vi "Dashboard Main.vi"() -> ()   [LabVIEW 2020]
uses:
  <vilib>/Utility/miscctls.llb/LVRectTypeDef.ctl
  <vilib>/event_ctls.llb/eventvkey.ctl
  <vilib>/Rock Robotics/WPI/DriverStation/WPI_DriverStationAllianceInfo.ctl
  <vilib>/Utility/miscctls.llb/LV3DPointTypeDef.ctl
  <vilib>/robotics/Kinematics/DH Kinematic Parameters.ctl
  <vilib>/robotics/Kinematics/Link/Joint Type.ctl
  b1c29fd4-b69e-4c47-bd92-218700034153.vi
  efc637a3-a7e0-4d6a-acb3-aee6468bd1cb.vi
  b2059994-562a-4507-8104-e4c00853bec9.vi
  7fc597ec-ac8e-4325-b133-71466b1fbbcb.vi
  9cac3b8b-4a3f-4d18-bfb1-3aae72e664f2.vi
  a7551b2b-ce58-4830-98e7-c5cf61f6feb4.vi
  cd51690b-7cbe-44fb-a5f0-3232adb0ed53.vi
  a4e8d5d1-2ec3-4e81-be0b-60391cc68073.vi
  dc64ebe6-91bd-4cd7-a1c2-6d709789b2ed.vi
  76b087ca-de3d-4263-8b5c-e25a6bef634b.vi
  1b78be80-bab2-445d-a3e8-82f142a16380.vi
  9e807339-2903-4f51-8fcc-64b6a9381567.vi
  e75f20ac-3dfa-4544-8614-4803d6d17fbb.vi
  273c17a0-a238-4f2a-a55a-7e29d73850ff.vi
  87bdd142-1820-4e26-8582-f713a5f3da40.vi
  b8451b18-7b16-4e07-a196-a1bebf8ce026.vi
  5d307e9f-edd0-4132-a387-09c5916d43b1.vi
  0137daef-9682-45ba-80b9-2d4fda8852b8.vi
  f6a63fab-964b-4051-8314-d4414a0a258c.vi
  90e0fe9d-42b1-4a72-a6c8-4b9d9b3a5a2a.vi
  f15e925d-3118-43e3-bf67-a1272bbf81dd.vi
  394886aa-4cdd-4740-8681-89e3e438764a.vi
  77a42c1f-99bf-4bb6-8218-45b49017f7dc.vi
  5abae45b-ab2b-4816-ba0c-2a0b218f6531.vi
  31f70c1d-3051-4c77-9544-a691198ba614.vi
  f63f5451-5db6-487e-bc86-5cb81e92b132.vi
  81d0db6a-d68a-45c3-b3b1-458879412541.vi
  c235c188-eb56-46fb-93d3-e8acf396af31.vi
  115ba94a-0b26-47fa-ae73-5ec5bd9e502a.vi
  2422668c-951b-48e5-9bda-0f59c56d9c0d.vi
  7776664e-4af7-4b3d-b288-2266642a045e.vi
  6004ed5d-dfc4-4dad-95c1-8e371ea2b9cd.vi
  321ce103-7778-4bb1-9ecc-75a76fef05e9.vi
  d30e88cc-5e2b-4867-b271-53fc6d5cd4d7.vi
  fde90579-e212-4b8a-8145-a17c3e40bcbd.vi
  6c63589b-432e-4f9c-bacb-2063ed7bd576.vi
  b7dcf304-99f6-4f78-9d14-19aa8d9ea562.vi
  e8b3bb93-ba91-445b-94c6-9e998421f827.vi
  0480a820-69ef-45e6-a9f4-d7ff60c89e45.vi
  1c99237e-ea3d-4ecf-b7c2-61034db3ecd2.vi
  58c381f4-7755-468c-a50e-7cea281bf291.vi
  4681331b-9a70-4b27-b9d4-a17199d3c64e.vi
  7eff148d-a456-4b5f-9b0b-1967e164dc83.vi
  7f162a9b-0cf5-4928-819b-a88ae877a425.vi
  748c1db2-33d9-4a44-b6de-b54d4bfa6e8e.vi
  0d2f8b8f-8dae-480e-9309-747785a3eba2.vi
  6da817f6-1561-45f8-a0fe-2c1e5adf6540.vi
  c02c89a6-b8c9-4f9c-9e24-ceb1b894960a.vi
  0a8fe2ab-d060-4915-a9b5-d8978247e2b6.vi
  b1c29fd4-b69e-4c47-bd92-218700034153.vi/77c742ae-e671-49bb-a825-a6e8cebc9f63.vi
  b2059994-562a-4507-8104-e4c00853bec9.vi/77c742ae-e671-49bb-a825-a6e8cebc9f63.vi
  9cac3b8b-4a3f-4d18-bfb1-3aae72e664f2.vi/77c742ae-e671-49bb-a825-a6e8cebc9f63.vi
  a7551b2b-ce58-4830-98e7-c5cf61f6feb4.vi/77c742ae-e671-49bb-a825-a6e8cebc9f63.vi
  cd51690b-7cbe-44fb-a5f0-3232adb0ed53.vi/77c742ae-e671-49bb-a825-a6e8cebc9f63.vi
  a4e8d5d1-2ec3-4e81-be0b-60391cc68073.vi/77c742ae-e671-49bb-a825-a6e8cebc9f63.vi
  dc64ebe6-91bd-4cd7-a1c2-6d709789b2ed.vi/77c742ae-e671-49bb-a825-a6e8cebc9f63.vi
  76b087ca-de3d-4263-8b5c-e25a6bef634b.vi/77c742ae-e671-49bb-a825-a6e8cebc9f63.vi
  1b78be80-bab2-445d-a3e8-82f142a16380.vi/77c742ae-e671-49bb-a825-a6e8cebc9f63.vi
  9e807339-2903-4f51-8fcc-64b6a9381567.vi/77c742ae-e671-49bb-a825-a6e8cebc9f63.vi
  e75f20ac-3dfa-4544-8614-4803d6d17fbb.vi/77c742ae-e671-49bb-a825-a6e8cebc9f63.vi
  0137daef-9682-45ba-80b9-2d4fda8852b8.vi/77c742ae-e671-49bb-a825-a6e8cebc9f63.vi
  f6a63fab-964b-4051-8314-d4414a0a258c.vi/77c742ae-e671-49bb-a825-a6e8cebc9f63.vi
  90e0fe9d-42b1-4a72-a6c8-4b9d9b3a5a2a.vi/77c742ae-e671-49bb-a825-a6e8cebc9f63.vi
  f15e925d-3118-43e3-bf67-a1272bbf81dd.vi/77c742ae-e671-49bb-a825-a6e8cebc9f63.vi
  394886aa-4cdd-4740-8681-89e3e438764a.vi/77c742ae-e671-49bb-a825-a6e8cebc9f63.vi
  77a42c1f-99bf-4bb6-8218-45b49017f7dc.vi/77c742ae-e671-49bb-a825-a6e8cebc9f63.vi
  5abae45b-ab2b-4816-ba0c-2a0b218f6531.vi/77c742ae-e671-49bb-a825-a6e8cebc9f63.vi
  31f70c1d-3051-4c77-9544-a691198ba614.vi/77c742ae-e671-49bb-a825-a6e8cebc9f63.vi
  f63f5451-5db6-487e-bc86-5cb81e92b132.vi/77c742ae-e671-49bb-a825-a6e8cebc9f63.vi
  81d0db6a-d68a-45c3-b3b1-458879412541.vi/77c742ae-e671-49bb-a825-a6e8cebc9f63.vi
  c235c188-eb56-46fb-93d3-e8acf396af31.vi/77c742ae-e671-49bb-a825-a6e8cebc9f63.vi
  115ba94a-0b26-47fa-ae73-5ec5bd9e502a.vi/77c742ae-e671-49bb-a825-a6e8cebc9f63.vi
  2422668c-951b-48e5-9bda-0f59c56d9c0d.vi/77c742ae-e671-49bb-a825-a6e8cebc9f63.vi
  7776664e-4af7-4b3d-b288-2266642a045e.vi/77c742ae-e671-49bb-a825-a6e8cebc9f63.vi
  6004ed5d-dfc4-4dad-95c1-8e371ea2b9cd.vi/77c742ae-e671-49bb-a825-a6e8cebc9f63.vi
  321ce103-7778-4bb1-9ecc-75a76fef05e9.vi/77c742ae-e671-49bb-a825-a6e8cebc9f63.vi
  d30e88cc-5e2b-4867-b271-53fc6d5cd4d7.vi/77c742ae-e671-49bb-a825-a6e8cebc9f63.vi
  fde90579-e212-4b8a-8145-a17c3e40bcbd.vi/77c742ae-e671-49bb-a825-a6e8cebc9f63.vi
  6c63589b-432e-4f9c-bacb-2063ed7bd576.vi/77c742ae-e671-49bb-a825-a6e8cebc9f63.vi
  b7dcf304-99f6-4f78-9d14-19aa8d9ea562.vi/77c742ae-e671-49bb-a825-a6e8cebc9f63.vi
  e8b3bb93-ba91-445b-94c6-9e998421f827.vi/77c742ae-e671-49bb-a825-a6e8cebc9f63.vi
  0480a820-69ef-45e6-a9f4-d7ff60c89e45.vi/77c742ae-e671-49bb-a825-a6e8cebc9f63.vi
  1c99237e-ea3d-4ecf-b7c2-61034db3ecd2.vi/77c742ae-e671-49bb-a825-a6e8cebc9f63.vi
  58c381f4-7755-468c-a50e-7cea281bf291.vi/77c742ae-e671-49bb-a825-a6e8cebc9f63.vi
  4681331b-9a70-4b27-b9d4-a17199d3c64e.vi/77c742ae-e671-49bb-a825-a6e8cebc9f63.vi
  7eff148d-a456-4b5f-9b0b-1967e164dc83.vi/77c742ae-e671-49bb-a825-a6e8cebc9f63.vi
  7f162a9b-0cf5-4928-819b-a88ae877a425.vi/77c742ae-e671-49bb-a825-a6e8cebc9f63.vi
  748c1db2-33d9-4a44-b6de-b54d4bfa6e8e.vi/77c742ae-e671-49bb-a825-a6e8cebc9f63.vi
  0d2f8b8f-8dae-480e-9309-747785a3eba2.vi/77c742ae-e671-49bb-a825-a6e8cebc9f63.vi
  <vilib>/robotics/Kinematics/RotateX.vi
  <vilib>/robotics/Kinematics/RotateY.vi
  <vilib>/robotics/Kinematics/RotateZ.vi
  <vilib>/Analysis/baseanly.llb/A x B.vi
  <vilib>/Analysis/baseanly.llb/Real A x B.vi
  0a8fe2ab-d060-4915-a9b5-d8978247e2b6.vi/77c742ae-e671-49bb-a825-a6e8cebc9f63.vi
  <vilib>/Utility/xml.llb/Read From XML File(array).vi
  <vilib>/Utility/xml.llb/Write to XML File(string).vi
  <vilib>/Rock Robotics/Network Tables/NT Read Number.vi
  <vilib>/Rock Robotics/Network Tables/NT Read Boolean.vi
  GlobalDashboard.vi
  <vilib>/Rock Robotics/Network Tables/NT Read String.vi
  <vilib>/Rock Robotics/Network Tables/NT Write Number.vi
  <vilib>/Rock Robotics/Network Tables/NT Read Numeric Array.vi
  <vilib>/Rock Robotics/Network Tables/NT Write Boolean.vi
  <vilib>/Rock Robotics/Network Tables/NT Read String Array.vi
  <vilib>/Rock Robotics/Network Tables/NT Read Boolean Array.vi
  <vilib>/Rock Robotics/Network Tables/NT Write String.vi
  <vilib>/Rock Robotics/Network Tables/NT Write Numeric Array.vi
  <vilib>/robotics/Kinematics/Analytical/Initialize Generic Serial Arm.vi
  <vilib>/picture/3D Picture Control/Object/Create Object (drawable).vi
  <vilib>/picture/3D Picture Control/Object/Add Object (no reference).vi
  <vilib>/Rock Robotics/Network Tables/NT Write String Array.vi
  <vilib>/vision/NI_Vision_Development_Module.lvlib
  <vilib>/picture/3D Picture Control/NI_3D Picture Control.lvlib
  <vilib>/robotics/Kinematics/Plotting/NI_Robotics_3DKinematics.lvlib
  <vilib>/robotics/Kinematics/Robot/NI_Robotics_Serial Robot Arm.lvclass
  <vilib>/robotics/Kinematics/Analytical/NI_Robotics_AnalyticKinematics.lvlib
  <vilib>/robotics/Kinematics/Link/NI_Robotics_Link.lvclass
  <vilib>/robotics/Kinematics/NI_Kinematics.lvlib
panel:
  in  "TCP":refnum<k5>
  in  "Dashboard Tab":T1(tab)=enum."Setup/Auto"
  in  "CheckList":i32(listbox)
  in  "Apply_Grid_Calibration":bool
  out "Current_Red_Calibration":dbl format="%.1f"
  in  "New_Red_Calibration":dbl format="%.1f"
  out "Heading_to_Target":dbl format="%.1f"
  out "Distance_to_Target":dbl format="%.1f"
  out "Robot_P":dbl format="%.1f"
  in  "Enable_Streaming_GUI":bool=TRUE
  out "Robot_Profile_GUI":string
  out "Auto_Playbook_GUI":string
  in  "Select Driver Profile":u16(ring) items=["N/A"]
  in  "Camera Name":string(combo)="limelight"
  in  "Camera Settings":T2={"Frame Rate"=20, "Compression"=60, "Size"=1, "DB Camera Config"=FALSE} {"Size" items=["640x480", "320x240", "160x120"]}
  in  "Select Autonomous Play":u16(ring) items=["N/A"]
  out "Master_Caution_GUI_0":bool caption="Mode_Butterfly"
  out "Robot_is_Autonomous_GUI_0":bool caption="Mode_Butterfly"
  out "Robot_Code_Version_GUI":string
  out "Auto_Suffix_GUI":string
  in  "Refresh_Auto_Play_List_GUI":bool
  in  "Auto_Delay_GUI":dbl format="%.1f"
  in  "Manual_Start_X":dbl min=0.0 max=700.0 format="%.1f"
  out "Robot_X":dbl format="%.1f"
  out "Robot_Y":dbl format="%.1f"
  in  "Manual_Start_Y":dbl min=0.0 max=400.0 format="%.1f"
  out "Robot_H_GUI":dbl format="%.1f"
  in  "Manual_Start_H":dbl min=0.0 max=360.0 format="%.1f"
  in  "Field Map":u16(ring) items=["N/A"]
  in  "Push_Robot_Start_GUI":bool
  in  "Export_Robot_Pose":bool
  in  "Clear_Robot_Pose_Display":bool
  in  "Dock_Dashboard":bool
  in  "Force_Human_Control_GUI":bool
  in  "Auto_Test_Mode_GUI":bool
  in  "Disable_Fusion_While_Autonomous":bool
  in  "Disable_Fusion_While_Disabled":bool=TRUE
  out "Robot Pose 1":cluster{dbl[], dbl[]}[](graph)
  in  "New_Blue_Calibration":dbl format="%.1f"
  out "Current_Blue_Calibration":dbl format="%.1f"
  in  "Scoring Position":u16(ring) items=["MID", "HIGH"]
  in  "TeleOp Starting State":u16(ring) items=["STOW", "GROUND"]
  out "Help Graphic":T3(plugin-control)
  out "Hybrid_Node_Names":bool
  out "Scored_Hybrid_Nodes":bool[](array[boolean])
  out "Nearest_Hybrid_Node":bool[](array[boolean])
  out "LL_Ret_Left":bool
  out "LL_Ret_Right":bool
  out "WA_Ret_Right":bool
  out "WA_Ret_Left":bool
  out "Gripper_Motor_Fault":bool
  out "Gripper_Overheating":bool
  out "Swerve_Drive_Fault":bool
  out "Arm_Motor_Over_Current":bool
  out "Arm_Motor_Fault":bool
  out "State_Score":bool
  out "State_Shelf":bool
  in  "Arm_Override":bool
  out "Score_State_LVL2_Indicator":bool
  out "Score_State_LVL1_Indicator":bool
  out "Arm_Overheating":bool
  out "Robot Pose 2":cluster{dbl[], dbl[]}[](graph)
  out "Master_State_SHLF_Indicator":bool
  out "Master_State_GRND_Indicator":bool
  out "Master_State_HOPR_Indicator":bool
  out "Master_State_SCOR_Indicator":bool
  out "Master_State_BLNC_Indicator":bool
  out "Master_State_STOW_Indicator":bool
  out "Vision_Fault_GUI":bool
  out "Pressure_Leak_GUI":bool
  in  "Master_Safety_Override_1":bool
  in  "Manipulator_Help":bool
  in  "Driver_Help":bool
  out "No_Secondary_Camera":bool
  out "Swerve_Shifter_Failure":bool
  out "Electrical_Fault_GUI":bool
  out "Diverting_Power_GUI":bool
  out "CAN_Bus_Fault_GUI":bool
  out "IMU_Failure_GUI":bool
  out "Robot_is_Autonomous_GUI_1":bool caption="Mode_Butterfly"
  out "LL_Valid":bool caption="Mode_Butterfly"
  out "Auto_Error_GUI":bool
  in  "Clear_Errors_GUI":bool
  out "Swerve_Azimuth_Fault":bool
  out "Pressure_Transducer_GUI":dbl(slide) scale=0.0..115.0
  out "Pressure_Vent_GUI":bool
  out "Swerve_Overheating":bool
  out "Compressor_On_GUI":bool
  in  "Right":bool
  in  "Reticule":T4(ring)
  in  "Save":bool
  in  "Up":bool
  in  "Down":bool
  in  "Left":bool
  out "Master_Caution_GUI_1":bool caption="Mode_Butterfly"
  out "Battery_Critical_GUI":bool
  out "Battery_Voltage_GUI":dbl(slide) scale=11.0..13.0
  out "Field_Oriented_GUI":bool caption="Mode_Butterfly"
  out "Slow_Loop":bool
  out "Combined Camera Feed":T3(plugin-control)
  in  "Camera_Override_GUI":bool
  in  "Field_Oriented_Override_GUI":bool
  out "Arm_Has_Arrived":bool caption="Mode_Butterfly"
  out "Pointed_at_Target":bool caption="Mode_Butterfly"
  in  "Auto_Targeting_Override":bool
  out "Arm_Motor_Fault_Array":bool[](array[boolean])
  out "Arm_Motor_Over_Current_Array":bool[](array[boolean])
  out "State_Hopper":bool
  out "Gripper_Outtaking":bool caption="Mode_Butterfly"
  out "Gripper_Intaking":bool caption="Mode_Butterfly"
  out "Gamepiece_Grabbed_1":bool caption="Mode_Butterfly"
  out "Using_Auto_Targeting":bool caption="Mode_Butterfly"
  out "Gripper_Velocity":dbl
  out "Swerve_Output_Loop_Time_GU":u32
  in  "Simulate_Arm":bool
  in  "Jog Z (in)":dbl min=-100.0 max=100.0 step=1.0 format="%.1g"
  in  "Unlock_Arm_Joints":bool
  out "Shoulder_Temp":dbl
  out "Ebow_Temp":dbl
  out "Wrist_Temp":dbl
  in  "Reset 3D View":bool
  out "Swerve_3_Drive_Velocity":dbl format="%.1f"
  out "Swerve_3_Azimuth_Position":dbl format="%.1f"
  out "Swerve_3_Drive_Temperature":dbl
  out "Swerve_0_Drive_Temperature":dbl
  out "Camera Perf":string
  out "Control_Loop_Time_GUI":u32
  in  "Calibrate_Wheels_GUI":bool
  in  "Home_Wheels_GUI":bool
  out "Swerve_0_Azimuth_Position":dbl format="%.1f"
  out "Swerve_0_Drive_Velocity":dbl format="%.1f"
  out "Swerve_1_Drive_Velocity":dbl format="%.1f"
  out "Swerve_1_Azimuth_Position":dbl format="%.1f"
  out "Swerve_1_Drive_Temperature":dbl
  out "Swerve_2_Drive_Velocity":dbl format="%.1f"
  out "Swerve_2_Azimuth_Position":dbl format="%.1f"
  out "Swerve_2_Drive_Temperature":dbl
  in  "Arm_Calibrate_Wheels_GUI":bool
  out "Master_Caution_GUI_2":bool caption="Mode_Butterfly"
  in  "Actuator Testing":u16(ring) items=["N/A"]
  in  "Test_Actuator_Value_GUI":dbl step=0.1 format="%.2f"
  in  "Calibrate_Joysticks_GUI":bool
  in  "Arm_Calibrate_Joysticks":bool
  out "Robot_is_Autonomous_GUI_2":bool caption="Mode_Butterfly"
  in  "Test_Actuator_Period_GUI":dbl min=0.0 step=1.0 format="%.2f"
  out "Pose_Loop_Time_GUI":u32
  in  "Mute_Audible_Warnings":bool
  out "Combined Error String":string
  out "Swerve_0_Shifter_State":string
  out "Swerve_1_Shifter_State":string
  out "Swerve_3_Shifter_State":string
  out "Swerve_2_Shifter_State":string
  out "Swerve_Azimuth_Fault_Array":bool[](array[boolean])
  in  "Super_Test_Mode_GUI":bool
  out "Current_Driver_Profile_Setpoints_GUI":T5={"Strafe Deadband"=0.08, "Strafe Scaling"=2.0, "Strafe Maximum"=0.5, "Rotation Deadband"=0.15, "Rotation Scaling"=2.5, "Rotation Maximum"=0.5} {"Rotation Maximum" min=0.3 max=1.0 scale=0.3..1.0; "Rotation Scaling" min=1.0 max=4.0 scale=1.0..4.0; "Rotation Deadband" min=0.0 max=0.25 scale=0.0..0.25; "Strafe Maximum" min=0.3 max=1.0 scale=0.3..1.0; "Strafe Scaling" min=1.0 max=4.0 scale=1.0..4.0; "Strafe Deadband" min=0.0 max=0.25 scale=0.0..0.25}
  in  "New_Driver_Profile_Setpoints_GUI":T6={"Strafe Deadband"=0.08, "Strafe Scaling"=2.0, "Strafe Max"=0.5, "Rotate Deadband"=0.15, "Rotate Scaling"=2.5, "Rotate Max"=0.5} {"Rotate Max" min=0.3 max=1.0 format="%.2g"; "Rotate Scaling" min=1.0 max=4.0 format="%.2g"; "Rotate Deadband" min=0.0 max=0.25 format="%.2g"; "Strafe Max" min=0.3 max=1.0 format="%.2g"; "Strafe Scaling" min=1.0 max=4.0 format="%.2g"; "Strafe Deadband" min=0.0 max=0.25 format="%.2g"}
  in  "Apply_Driver_Profile_Setpoints_GUI":bool
  out "Current_Driver_Profile_GUI":string
  in  "Free_Tuning_Variable_GUI":dbl min=0.0 step=1.0 format="%.3f"
  out "Audible_Warnings_Enabled_GUI":bool
  out "Legal_Drivers_GUI":string[](array[string])
  out "Swerve_Shifter_Failure_Array":bool[](array[boolean])
  out "Swerve_Overheating_Array":bool[](array[boolean])
  out "3D Arm Model":refnum<vi>(3d-picture)
  out "Shoulder_Current_Angle":dbl format="%.1f"
  out "Ebow_Current_Angle":dbl format="%.1f"
  out "Wrist_Current_Angle":dbl format="%.1f"
  out "Arm_Overheating_Array":bool[](array[boolean])
  out "Grabbed_Gamepiece_Enum":enum16{"CUBE", "CONE"}(ring)
  in  "Calibrate_Arm":bool
  in  "Arm_Calibrate_Arm":bool
  in  "Jog X (in)":dbl min=-100.0 max=100.0 step=1.0 format="%.1g"
  out "Gamepiece_Grabbed_2":bool caption="Mode_Butterfly"
  out "End_Effector_X":dbl format="%.1f"
  out "End_Effector_Z":dbl format="%.1f"
  out "Swerve_Drive_Fault_Array":bool[](array[boolean])
  out "Gripper_Temperature":dbl
  out "NT Connection":bool
  out "Mode":T7(ring)=enum."Auto Disabled"
  out "Tree":string(tree)
  out "Background":bool
  # "2023 Dashboard v2.3-dev"
  # "Robot Profile"
  # "Robot X Position (in)"
  # "Robot Y Position (in)"
  # "Delay (s)"
  # "Suffix"
  # "X (in)"
  # "Robot Heading (deg)"
  # "Autonomous Playbook Entry"
  # "Robot Pitch (deg)"
  # "Auto Test\nMode"
  # "Force\nHuman"
  # "Y (in)"
  # "Target Distance (in)"
  # "H (deg)"
  # "Target Heading (deg)"
  # "Undock Dashboard"
  # "Yes Camera Streaming"
  # "Stop Fusion While Auto"
  # "Stop Fusion While Disabled"
  # "Grid Y Calibration (in)"
  # "X"
  # "Y"
  # "MASTER\nSTATES"
  # "OVERRIDES"
  # "Camera Override"
  # "Robot-Oriented Drive Controls"
  # "Arm Motion Override"
  # "Auto-Targeting Override"
  # "SCORE\nSTATES"
  # "Disengage\nSafeties"
  # "11"
  # "13"
  # "0"
  # "120"
  # "Drivebase Subsytem"
  # "Arm and Gripper Subsytems"
  # "Driver Profile Selected"
  # "Calibrate Arm Encoders"
  # "Loop Times"
  # "Module 1"
  # "Module 0"
  # "Control (ms)"
  # "Azimuth (deg)"
  # "Pose (ms)"
  # "Temp (C)"
  # "Simulate the Arm"
  # "Unlock Arm Joints"
  # "Drive Output (ms)"
  # "Velocity (ft/s)"
  # "Shifter State"
  # "Module 2"
  # "Module 3"
  # "Variable (bleh)"
  # "Disabled\nTest Mode"
  # "Azimuth (deg)"
  # "Temp (C)"
  # "Velocity (ft/s)"
  # "Shifter State"
  # "Calibrate Wheels"
  # "Gripper"
  # "Shoulder"
  # "Elbow"
  # "Wrist"
  # "Period (s)"
  # "Calibrate Joysticks"
  # "Amplitude"
  # "Relative (deg)"
  # "Velocity (rpm)"
  # "Temp (C)"
  # "Temp (C)"
  # "0"
  # "0.25"
  # "1"
  # "4"
  # "0.3"
  # "1"
  # "0"
  # "0.25"
  # "1"
  # "4"
  # "0.3"
  # "1"
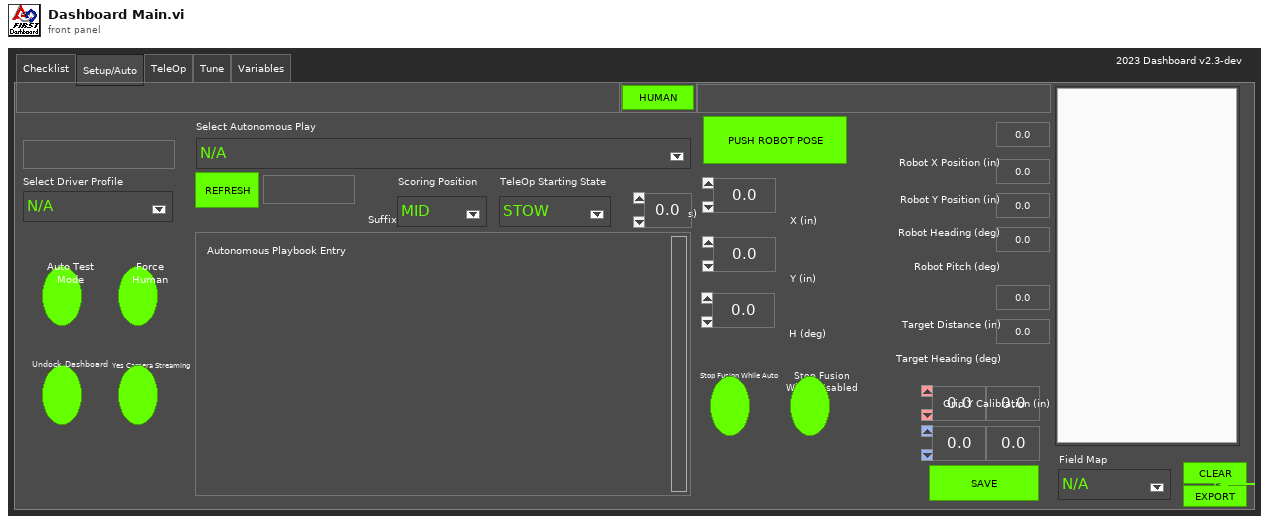
[diagram p1: front panel]
types:
  T1 = enum32{"Checklist", "Setup/Auto", "TeleOp", "Tune", "NT", "Test", "Commands", "Variables"}
  T2 = cluster{"Frame Rate":i32, "Compression":i32, "Size":u16, "DB Camera Config":bool}
  T3 = typedef "IMAQ Image.ctl" = refnum<image>
  T4 = enum16{"Wide Angle Left Reticule", "Wide Angle Right Reticule", "Lime Light Left Reticule", "Lime Light Right Reticule"}
  T5 = cluster{"Strafe Deadband":dbl, "Strafe Scaling":dbl, "Strafe Maximum":dbl, "Rotation Deadband":dbl, "Rotation Scaling":dbl, "Rotation Maximum":dbl}
  T6 = cluster{"Strafe Deadband":dbl, "Strafe Scaling":dbl, "Strafe Max":dbl, "Rotate Deadband":dbl, "Rotate Scaling":dbl, "Rotate Max":dbl}
  T7 = enum8{"Tele-Op Disabled", "Tele-Op Enabled", "Auto Disabled", "Auto Enabled", "Test Disabled", "Test Enabled", "Disconnected", "No Code", "E-Stop"}
  T8 = cluster{"Save Path":path, "Interval (s)":dbl, "Keep":i32}
  T9 = enum32{"Drive", "Camera", "Basic", "Custom", "Test", "Commands", "Checklist", "Variables"}
  T10 = cluster{"IDs":cluster{"RPC field ID":u16, "Unique ID":u16}, "String":string}
  T11 = typedef "Image Type" = u32
  T12 = typedef "WPI_DriverStationAllianceInfo.ctl" = enum16{"Red", "Blue", "Invalid"}
  T13 = typedef "LV3DPointTypeDef.ctl" = cluster{"X":sgl, "Y":sgl, "Z":sgl}
  T14 = cluster{"Red":sgl, "Green":sgl, "Blue":sgl, "Alpha":sgl}
  T15 = enum8{"Enabled", "Disabled", "Disabled and Grayed Out"}
  T16 = cluster{"Error Strings":string, "Disable Counts":cluster{u16, u16}, "Rail Faults":cluster{u16, u16, u16}, "Robot IP":string, "DB Mode":u8, "Event Info":cluster{"Name":string, "Type":u8, "Number":u16, "Replay":u8}}
  T17 = cluster{"Storage":cluster{"Disk Free":u64, "RAM Block":u32, "RAM free":u32}, "CPU Utilization":cluster{"CPU % ISR":sgl, "CPU % Time Crit":sgl, "CPU % Timed Str":sgl, "CPU % High":sgl, "CPU % Above":sgl, "CPU % Normal":sgl, "CPU % Low":sgl}, "CAN":cluster{"% Bus Utilization":sgl, "Bus Off Cnt":u32, "TX_FIFO Full Cnt":u32, "Receive Error Cnt":u8, "Transmit Error Cnt":u8}, "HID":cluster{"HID Outputs":u32, "Rumble Low":u16, "Rumble High":u16}[]}
  T18 = cluster{"Status bits":cluster{"Test Mode":bool, "Autonomous":bool, "Enabled":bool, "Code Start":bool, "Brownout":bool, "Reserved 2":bool, "Reserved 3":bool, "E-Stop":bool}, "Code Trace":cluster{"Disabled":bool, "TeleOp":bool, "Auto":bool, "Test":bool}, "Controller Type":enum16{"unknown", "cRIO", "roboRio"}, "Code?":enum16{"unknown", "noCode", "code"}, "Battery V":dbl}
  T19 = cluster{"Control Bits":cluster{"TestMode":bool, "Autonomous":bool, "Enabled":bool, "FMS Present":bool, bool, bool, bool, "E-Stop":bool}, "Team Station ":u8, "Countdown":sgl, "Joystick Values":cluster{"Axes":dbl[], "Buttons":bool[], "POVs":i16[]}[]}
  T20 = typedef "imagedata.ctl" = cluster{"image type":i32, "image depth":i32, "image":u8[], "mask":u8[], "colors":u32[], "Rectangle":cluster{"left":i16, "top":i16, "right":i16, "bottom":i16}}
  T21 = cluster{"Boolean":bool, "Numeric Text.Text Colors:Text Color":u32}
  T22 = cluster{"value[0]":dbl, "value[1]":dbl, "value[2]":dbl, "value[3]":dbl, "value[4]":dbl, "value[5]":dbl}
  T23 = typedef "DH Kinematic Parameters.ctl" = cluster{"twist angle":dbl, "length":dbl, "rotation angle":dbl, "offset distance":dbl, "joint type":T24, "joint coordinate offset":dbl}
  T24 = typedef "NI_Robotics_Link.lvclass/Joint Type.ctl" = enum16{"Revolute", "Prismatic"}
  T25 = typedef "NI_Matrix.lvlib/RealMatrix.ctl" = dbl[][]
  T26 = cluster{"Numeric":dbl, "Numeric":dbl, "Numeric":dbl}
  T27 = typedef "LVRectTypeDef.ctl" = cluster{"Left":i16, "Top":i16, "Right":i16, "Bottom":i16}
  T28 = typedef "eventvkey.ctl" = enum16{"ASCII", "Enter", "Return", "Shift", "Ctrl", "Alt", "Cmd", "Opt", "Caps", "NumLock", "Clear", "Break", "Up", "Down", "Left", "Right", "Insert", "Delete", "Home", "End", "PageUp", "PageDown", "Escape", "Help", "Pause", "ScrollLock", "F1", "F2", "F3", "F4", "F5", "F6", "F7", "F8", "F9", "F10", "F11", "F12", "F13", "F14", "F15", "F16", "F17", "F18", "F19", "F20", "F21", "F22", "F23", "F24", "Play", "VolumeUp", "VolumeDown", "Mute", "Two Byte Char"}
  T29 = cluster{"Shift":bool, "Ctrl":bool, "Alt":bool, "Cmd":bool, "Opt":bool}
  T30 = cluster{"WA_Ret_Left":refnum<vi>, "WA_Ret_Right":refnum<vi>, "LL_Ret_Left":refnum<vi>, "LL_Ret_Right":refnum<vi>}
  T31 = cluster{"Camera Name":string, string, "Saved DB Images Info":cluster{"Save Path":path, "Interval (s)":dbl, "Keep":i32}}
  T32 = cluster{string, "Arm_Motor_Over_Current":bool, dbl}
  T33 = cluster{string, "Swerve_Shifter_Failure":bool, dbl}
  T34 = cluster{string, "Master_Safety_Override_1":bool, dbl}
  T35 = cluster{string, "Swerve_Azimuth_Fault":bool, dbl}
  T36 = cluster{string, "Arm_Calibrate_Wheels_GUI":bool, dbl}
  T37 = cluster{string, "Electrical_Fault_GUI":bool, dbl}
  T38 = cluster{string, "Arm_Calibrate_Joysticks":bool, dbl}
  T39 = cluster{string, "Gripper_Motor_Fault":bool, dbl}[]
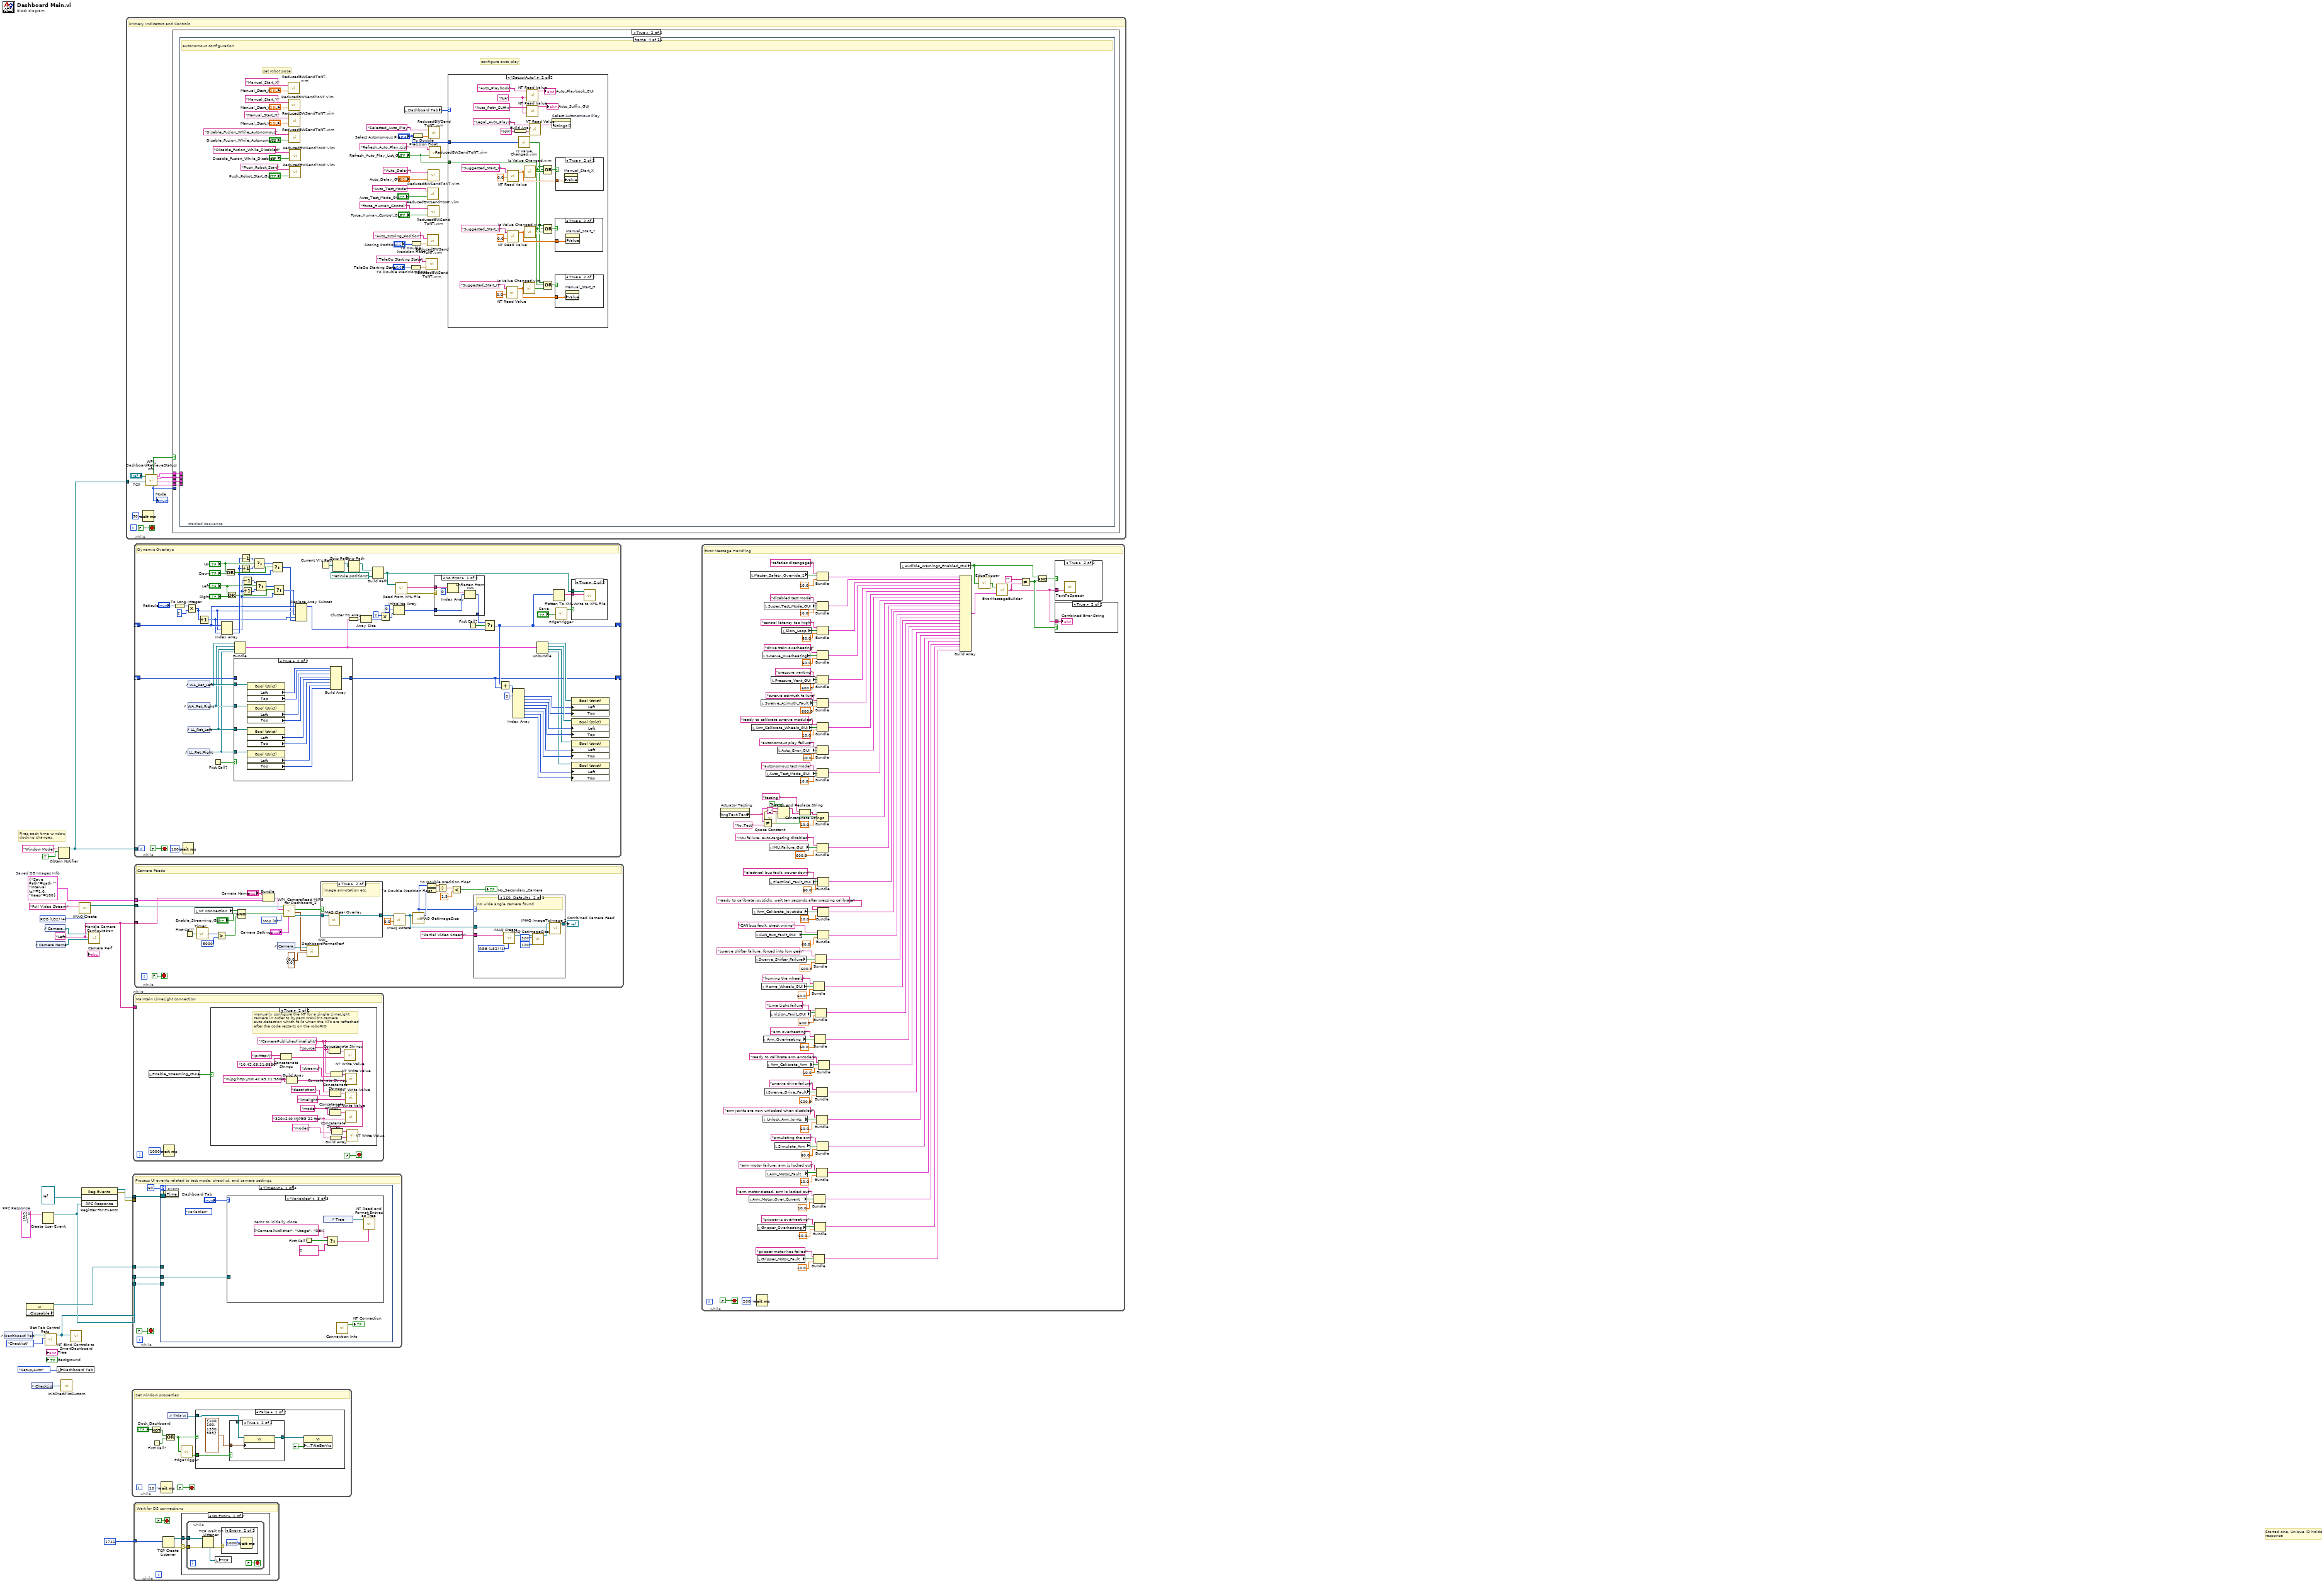
[diagram p0: block diagram]
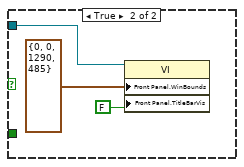
[diagram p4: hidden frame]
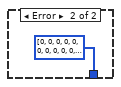
[diagram p7: hidden frame]
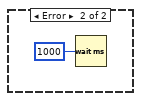
[diagram p11: hidden frame]
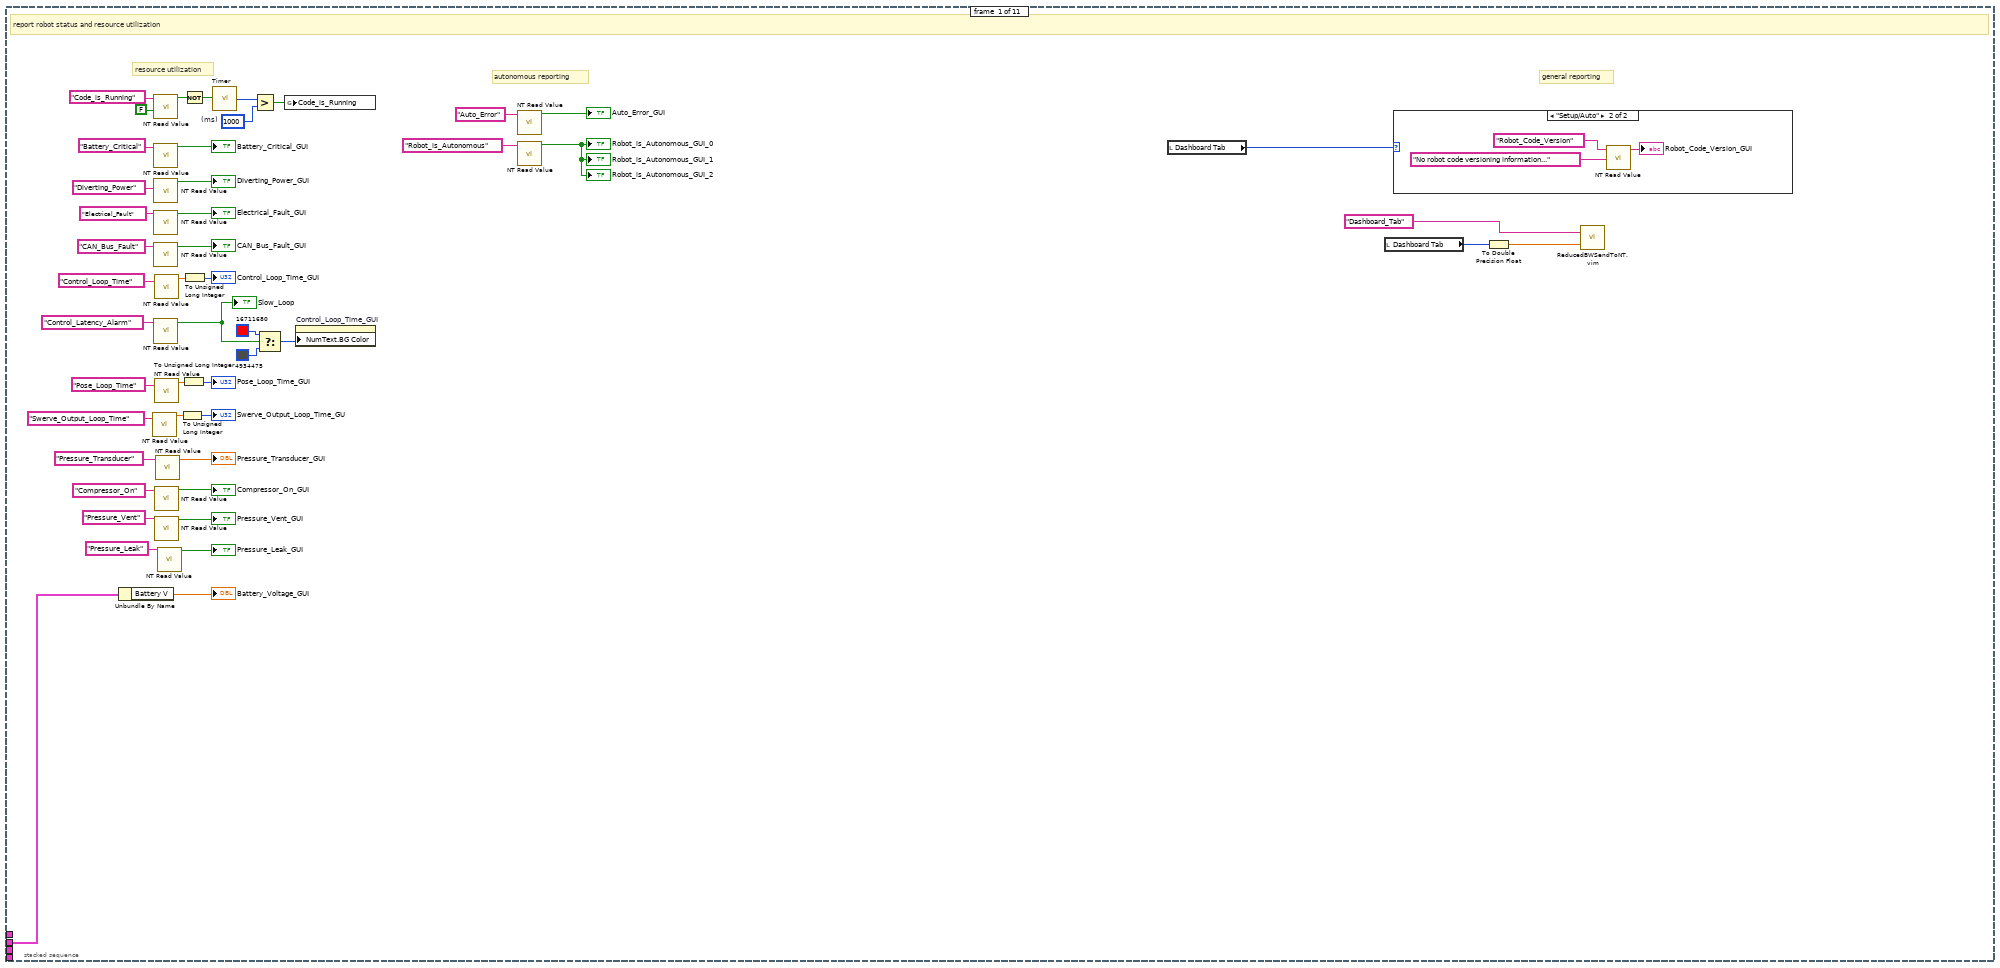
[diagram p13: hidden frame]
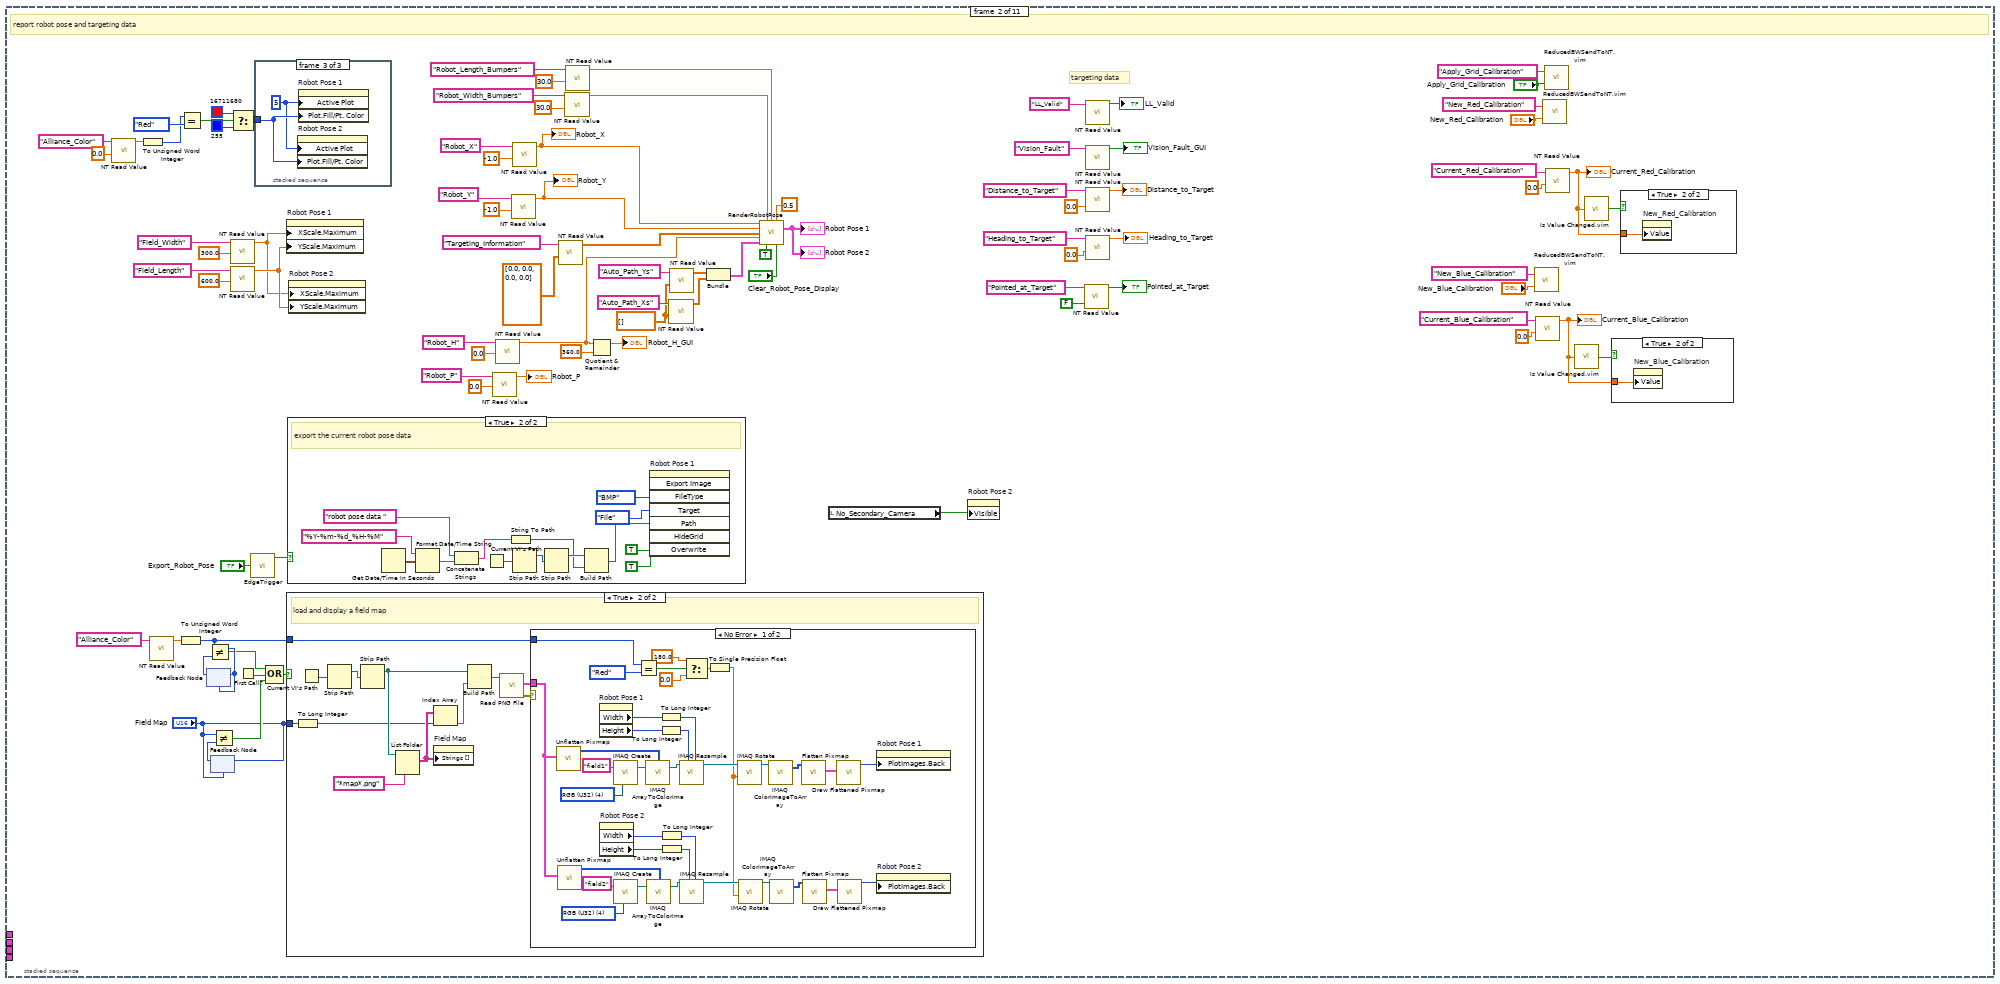
[diagram p15: hidden frame]
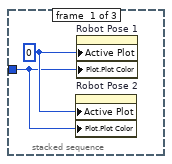
[diagram p18: hidden frame]
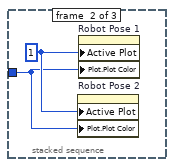
[diagram p19: hidden frame]
diagram:
  w10 = T8 {"Save Path"=path "", "Interval (s)"=1.0, "Keep"=180}  # Saved DB Images Info
  w3 = "Left"
  w13 = T10 {"IDs"={"RPC field ID"=0, "Unique ID"=0}, "String"=""}  # RPC Response
  w6 = T11 4 items=["Grayscale (U8)", "Grayscale (I16)", "Grayscale (SGL)", "Complex (CSG)", "RGB (U32)", "HSL (U32)", "RGB (U64)"] ("Image Type")
  # "Started one, Unique ID holds\nresponse"
  # "Fires each time window\ndocking changes."
  n1 = control-ref of="Dashboard Tab"() -> (w16:refnum<vi>)
  n2 = property class="VI" props=["Front Panel.Closeable"]() -> (reference out=w17:refnum<vi>)  [unwired: 2 in, 2 out]
  n3 = control-ref of="CheckList"() -> (w5:refnum<vi>)
  n4 = control-ref of="Camera Name"() -> (w8:refnum<vi>)
  n5 = Create User Event(user event datatype=w13) -> (user event=w12:refnum<user-event>)  [unwired: 1 in, 1 out]
  n6 = control-ref of="Camera Settings"() -> (w9:refnum<vi>)
  n7 = call <vilib>:"Get Tab Control Refs.vi"("Page Index"=T9."Checklist" ("Dashboard Tab"), "TabControl in"=w16) -> ("ControlsOnPage"=w2:refnum<vi>[])  [unwired: 9 in]
  n8 = local write "Dashboard Tab"(T1."Setup/Auto" ("Dashboard Tab")) -> ()
  n9 = Obtain Notifier(name (unnamed)="Window Mode", notification data type=TRUE) -> (notifier out=w1:refnum<notifier>)  [unwired: 2 in, 2 out]
  n10 = call "InitChecklistCustom.vi"("ListBox in"=w5) -> ()  [unwired: 1 in]
  n11 = call <vilib>:"NT Bind Controls to SmartDashboard.vi"("Bound Control Refs"=w2) -> ()  [unwired: 11 in]
  n12 = call "IMAQ Create"("Image Name"="Full Video Stream", "Image Type"=w6) -> ("New Image"=w4:T3)  [unwired: 2 in, 2 out]
  n13 = register-events(refnum<vi> refnum, w12) -> (reference out=w20:refnum<event-registration>, error out=w19:errorcluster)  [unwired: 2 in]
  n14 = call "Handle Camera Configuration.vi"("CameraNameRef"=w8, "Display Name"=w3, "ClusterRef"=w9) -> ()  [unwired: 9 in]
  n15 = while {
    tunnel: w1 -> [w24]
    stop <- FALSE stop-if-true
    # "Primary Indicators and Controls"
    n16 = Wait (ms)(milliseconds to wait=u32 50) -> ()  [unwired: 1 out]
    n17 = call <vilib>:"WPI_DashboardRetrieveStatusInfo.vi"("Window Mode Notifier"=w24, "TCP Cnx"="TCP") -> ("Power and Errors"=w27:T16, "Robot Metrics"=w30:T17, "Status Info"=w31:T18, "Control Info"=w28:T19, "Robot Mode"=w26:T7, "Process?"=w29:bool)  [unwired: 4 in]
    "Mode" <- w26
    n18 = case shown="True" w29 {
      tunnel: w31 -> [_ w35]
      tunnel: w30 -> [_ w34]
      tunnel: w28 -> [_ w36]
      tunnel: w27 -> [_ w33]
      tunnel: w26 -> [_ _]
      frame False {
      }
      frame True {
        n19 = stacked-sequence {
          tunnel: w36 -> [_ _ _ _ _ _ _ _ _ _ _]
          tunnel: w35 -> [w51 _ _ _ _ _ _ _ _ _ _]
          tunnel: w34 -> [_ _ _ _ _ _ _ _ _ _ _]
          tunnel: w33 -> [_ _ _ _ _ _ _ _ _ _ _]
          frame #0 {
            w41 = u32 1000  # (ms)
            # "general reporting"
            # "resource utilization"
            # "autonomous reporting"
            # "report robot status and resource utilization"
            n20 = Unbundle By Name(w51) -> ("Battery V"=→"Battery_Voltage_GUI":dbl)
            n21 = call-poly <vilib>:"NT Read Value.vi"("name"="Swerve_Output_Loop_Time" ("Name")) -> ("value"=w39:dbl)  [unwired: 8 in, 2 out]
            n22 = call-poly <vilib>:"NT Read Value.vi"("default value"=FALSE, "name"="Code_is_Running" ("Name")) -> ("value"=w44:bool)  [unwired: 7 in, 2 out]
            n23 = call-poly <vilib>:"NT Read Value.vi"("name"="Battery_Critical" ("Name")) -> ("value"=→"Battery_Critical_GUI":bool)  [unwired: 8 in, 2 out]
            n24 = call-poly <vilib>:"NT Read Value.vi"("name"="Diverting_Power" ("Name")) -> ("value"=→"Diverting_Power_GUI":bool)  [unwired: 8 in, 2 out]
            n25 = call-poly <vilib>:"NT Read Value.vi"("name"="Electrical_Fault" ("Name")) -> ("value"=→"Electrical_Fault_GUI":bool)  [unwired: 8 in, 2 out]
            n26 = call-poly <vilib>:"NT Read Value.vi"("name"="CAN_Bus_Fault" ("Name")) -> ("value"=→"CAN_Bus_Fault_GUI":bool)  [unwired: 8 in, 2 out]
            n27 = call-poly <vilib>:"NT Read Value.vi"("name"="Control_Latency_Alarm" ("Name")) -> ("value"=w80:bool)  [unwired: 8 in, 2 out]
            "Slow_Loop" <- w80
            n28 = call-poly <vilib>:"NT Read Value.vi"("name"="Control_Loop_Time" ("Name")) -> ("value"=w71:dbl)  [unwired: 8 in, 2 out]
            n29 = call-poly <vilib>:"NT Read Value.vi"("name"="Pose_Loop_Time" ("Name")) -> ("value"=w81:dbl)  [unwired: 8 in, 2 out]
            n30 = call-poly <vilib>:"NT Read Value.vi"("name"="Compressor_On" ("Name")) -> ("value"=→"Compressor_On_GUI":bool)  [unwired: 8 in, 2 out]
            n31 = call-poly <vilib>:"NT Read Value.vi"("name"="Pressure_Vent" ("Name")) -> ("value"=→"Pressure_Vent_GUI":bool)  [unwired: 8 in, 2 out]
            n32 = call-poly <vilib>:"NT Read Value.vi"("name"="Pressure_Transducer" ("Name")) -> ("value"=→"Pressure_Transducer_GUI":dbl)  [unwired: 8 in, 2 out]
            n33 = call-poly <vilib>:"NT Read Value.vi"("name"="Pressure_Leak" ("Name")) -> ("value"=→"Pressure_Leak_GUI":bool)  [unwired: 8 in, 2 out]
            n34 = To Unsigned Long Integer(number=w39) -> (unsigned 32bit integer=→"Swerve_Output_Loop_Time_GU":u32)
            n35 = To Unsigned Long Integer(number=w81) -> (unsigned 32bit integer=→"Pose_Loop_Time_GUI":u32)
            n36 = Not(x=w44) -> (.not. x?=w43:bool)
            n37 = To Unsigned Long Integer(number=w71) -> (unsigned 32bit integer=→"Control_Loop_Time_GUI":u32)
            n38 = call "Timer.vi"("Reset Timer"=w43) -> ("Time (ms)"=w42:u32)
            n39 = Greater?(x=w42, y=w41) -> (0:w40:bool)
            n40 = Select(t=u32 16711680 ("Numeric Text.Text Colors:Text Color"), s=w80, f=u32 4934475 ("Numeric Text.Text Colors:Text Color")) -> (s? t:f=w75:u32)
            n41 = global write "GlobalDashboard.vi" "Code_is_Running"(w40) -> ()
            n42 = property on="Control_Loop_Time_GUI" class="DigNum (strict)"("NumText.BG Color"=w75) -> ()  [unwired: 2 in, 2 out]
            n43 = call-poly <vilib>:"NT Read Value.vi"("name"="Auto_Error" ("Name")) -> ("value"=→"Auto_Error_GUI":bool)  [unwired: 8 in, 2 out]
            n44 = call-poly <vilib>:"NT Read Value.vi"("name"="Robot_is_Autonomous" ("Name")) -> ("value"=→"Robot_is_Autonomous_GUI_0" →"Robot_is_Autonomous_GUI_1" →"Robot_is_Autonomous_GUI_2":bool)  [unwired: 8 in, 2 out]
            n45 = local read "Dashboard Tab"() -> (w47:T1)
            n46 = local read "Dashboard Tab"() -> (w48:T1)
            n47 = case shown="\"Setup/Auto\"" w47 {
              frame "Checklist", Default {
              }
              frame "Setup/Auto" {
                n48 = call-poly <vilib>:"NT Read Value.vi"("default value"="No robot code versioning information..." ("Default Value"), "name"="Robot_Code_Version" ("Name")) -> ("value"=→"Robot_Code_Version_GUI":string)  [unwired: 7 in, 2 out]
              }
            }
            n49 = To Double Precision Float(number=w48) -> (double precision float=w49:dbl)
            n50 = call "ReducedBWSendToNT.vim"("Value In"=w49, "NT Name"="Dashboard_Tab" ("Name")) -> ()  [unwired: 1 out]
          }
          frame #1 {
            w87 = dbl[] [] ("default value")
            # "targeting data"
            # "report robot pose and targeting data"
            n51 = call-poly <vilib>:"NT Read Value.vi"("default value"=0.0, "name"="Alliance_Color" ("Name")) -> ("value"=w131:dbl)  [unwired: 7 in, 2 out]
            n52 = To Unsigned Word Integer(number=w131) -> (unsigned 16bit integer=w129:u16)
            n53 = call-poly <vilib>:"NT Read Value.vi"("name"="Alliance_Color" ("Name")) -> ("value"=w149:dbl)  [unwired: 8 in, 2 out]
            n54 = To Unsigned Word Integer(number=w149) -> (unsigned 16bit integer=w159:u16)
            n55 = Equal?(x=w129, y=WPI_DriverStationAllianceInfo."Red" ("x")) -> (x = y?=w122:bool)
            n56 = feedback #1(w159) -> (w155:u16)
            n57 = feedback-in #1(w159) -> ()
            n58 = Not Equal?(x=w159, y=w155) -> (x != y?=w157:bool)
            n59 = feedback #2("Field Map") -> (w160:u16)
            n60 = feedback-in #2("Field Map") -> ()
            n61 = Not Equal?(x="Field Map", y=w160) -> (x != y?=w162:bool)
            n62 = call-poly <vilib>:"NT Read Value.vi"("default value"=300.0 ("Default Value"), "name"="Field_Width" ("Name")) -> ("value"=w123:dbl)  [unwired: 7 in, 2 out]
            n63 = call-poly <vilib>:"NT Read Value.vi"("default value"=600.0 ("Default Value"), "name"="Field_Length" ("Name")) -> ("value"=w124:dbl)  [unwired: 7 in, 2 out]
            n64 = Select(t=u32 16711680 ("Color"), s=w122, f=u32 255 ("Color")) -> (s? t:f=w125:u32)
            n65 = First Call?() -> (First Call?: T/F=w156:bool)
            n66 = call "EdgeTrigger.vi"("Input Signal"="Export_Robot_Pose") -> ("Rising Edge Trigger"=w163:bool)  [unwired: 2 out]
            n67 = stacked-sequence {
              tunnel: w125 -> [w177 w179 w182]
              frame #0 {
                w178 = u32 0 ("Active Plot")
                n68 = property on="Robot Pose 2" class="XYGraph (strict)"("Active Plot"=w178, "Plot.Plot Color"=w177) -> ()  [unwired: 2 in, 2 out]
                n69 = property on="Robot Pose 1" class="XYGraph (strict)"("Active Plot"=w178, "Plot.Plot Color"=w177) -> ()  [unwired: 2 in, 2 out]
              }
              frame #1 {
                w180 = u32 1 ("Active Plot")
                n70 = property on="Robot Pose 2" class="XYGraph (strict)"("Active Plot"=w180, "Plot.Plot Color"=w179) -> ()  [unwired: 2 in, 2 out]
                n71 = property on="Robot Pose 1" class="XYGraph (strict)"("Active Plot"=w180, "Plot.Plot Color"=w179) -> ()  [unwired: 2 in, 2 out]
              }
              frame #2 {
                w181 = u32 5 ("Active Plot")
                n72 = property on="Robot Pose 2" class="XYGraph (strict)"("Active Plot"=w181, "Plot.Fill/Pt. Color"=w182) -> ()  [unwired: 2 in, 2 out]
                n73 = property on="Robot Pose 1" class="XYGraph (strict)"("Active Plot"=w181, "Plot.Fill/Pt. Color"=w182) -> ()  [unwired: 2 in, 2 out]
              }
            }
            n74 = Compound Arithmetic op=OR(w157, w156, w162) -> (w158:bool)
            n75 = property on="Robot Pose 1" class="XYGraph (strict)"("XScale.Maximum"=w123, "YScale.Maximum"=w124) -> ()  [unwired: 2 in, 2 out]
            n76 = case shown="True" w158 {
              tunnel: w159 -> [_ w189]
              tunnel: "Field Map" -> [_ w187]
              frame False {
              }
              frame True {
                # "load and display a field map"
                n77 = To Long Integer(number=w187) -> (32bit integer=w185:i32)
                n78 = Current VI's Path() -> (path=w192:path)
                n79 = Strip Path(path=w192) -> (stripped path=w191:path)  [unwired: 1 out]
                n80 = Strip Path(path=w191) -> (stripped path=w188:path)  [unwired: 1 out]
                n81 = List Folder(path=w188, pattern="*map*.png") -> (filenames=w186:string[])  [unwired: 2 in, 3 out]
                n82 = Index Array(array=w186, index=w185) -> (element=w184:string)
                n83 = property on="Field Map" class="Ring (strict)"("Strings []"=w186) -> ()  [unwired: 2 in, 2 out]
                n84 = Build Path(base path=w188, name or relative path=w184) -> (appended path=w190:path)
                n85 = call <vilib>:"Read PNG File.vi"("path to PNG file"=w190) -> ("error out"=w194:errorcluster, "image data"=w193:T20)  [unwired: 8 in, 1 out]
                n86 = case shown="No Error" w194 {
                  tunnel: w193 -> [w197 _]
                  tunnel: w189 -> [w212 _]
                  frame No Error {
                    w207 = T11 4 items=["Grayscale (U8)", "Grayscale (I16)", "Grayscale (SGL)", "Complex (CSG)", "RGB (U32)", "HSL (U32)", "RGB (U64)", "Grayscale (U16)"] ("Image Type")
                    w227 = T11 4 items=["Grayscale (U8)", "Grayscale (I16)", "Grayscale (SGL)", "Complex (CSG)", "RGB (U32)", "HSL (U32)", "RGB (U64)", "Grayscale (U16)"] ("Image Type")
                    n87 = call <vilib>:"Unflatten Pixmap.vi"("image data"=w197) -> ("24-bit pixmap"=w226:u32[][])  [unwired: 4 in, 6 out]
                    n88 = call <vilib>:"Unflatten Pixmap.vi"("image data"=w197) -> ("24-bit pixmap"=w206:u32[][])  [unwired: 4 in, 6 out]
                    n89 = property on="Robot Pose 1" class="XYGraph (strict)"() -> ("Width"=w230:u32, "Height"=w229:u32)  [unwired: 2 in, 2 out]
                    n90 = property on="Robot Pose 2" class="XYGraph (strict)"() -> ("Width"=w210:u32, "Height"=w209:u32)  [unwired: 2 in, 2 out]
                    n91 = call "IMAQ Create"("Image Name"="field1", "Image Type"=w227) -> ("New Image"=w225:T3)  [unwired: 3 in, 1 out]
                    n92 = call "IMAQ Create"("Image Name"="field2", "Image Type"=w207) -> ("New Image"=w205:T3)  [unwired: 3 in, 1 out]
                    n93 = Equal?(x=w212, y=WPI_DriverStationAllianceInfo."Red" ("x")) -> (x = y?=w214:bool)
                    n94 = call "IMAQ ArrayToColorImage"("Image Pixels (U32)"=w226, "Image"=w225) -> ("Image Out"=w224:T3)  [unwired: 3 in, 1 out]
                    n95 = call "IMAQ ArrayToColorImage"("Image Pixels (U32)"=w206, "Image"=w205) -> ("Image Out"=w204:T3)  [unwired: 3 in, 1 out]
                    n96 = To Long Integer(number=w230) -> (32bit integer=w220:i32)
                    n97 = To Long Integer(number=w229) -> (32bit integer=w221:i32)
                    n98 = To Long Integer(number=w210) -> (32bit integer=w200:i32)
                    n99 = To Long Integer(number=w209) -> (32bit integer=w201:i32)
                    n100 = call "IMAQ Resample"("X Resolution"=w220, "Y Resolution"=w221, "Image Src"=w224) -> ("Image Dst Out"=w219:T3)  [unwired: 7 in, 1 out]
                    n101 = call "IMAQ Resample"("X Resolution"=w200, "Y Resolution"=w201, "Image Src"=w204) -> ("Image Dst Out"=w199:T3)  [unwired: 7 in, 1 out]
                    n102 = Select(t=180.0, s=w214, f=0.0) -> (s? t:f=w217:dbl)
                    n103 = To Single Precision Float(number=w217) -> (single precision float=w195:sgl)
                    n104 = call "IMAQ Rotate"("Angle (degrees)"=w195, "Image Src"=w219) -> ("Image Dst Out"=w218:T3)  [unwired: 8 in, 1 out]
                    n105 = call "IMAQ Rotate"("Angle (degrees)"=w195, "Image Src"=w199) -> ("Image Dst Out"=w198:T3)  [unwired: 8 in, 1 out]
                    n106 = call "IMAQ ColorImageToArray"("Image"=w218) -> ("Image Pixels (U32)"=w223:u32[][])  [unwired: 3 in, 2 out]
                    n107 = call "IMAQ ColorImageToArray"("Image"=w198) -> ("Image Pixels (U32)"=w203:u32[][])  [unwired: 3 in, 2 out]
                    n108 = call <vilib>:"Flatten Pixmap.vi"("24-bit pixmap"=w223) -> ("image data"=w222:T20)  [unwired: 10 in]
                    n109 = call <vilib>:"Flatten Pixmap.vi"("24-bit pixmap"=w203) -> ("image data"=w202:T20)  [unwired: 10 in]
                    n110 = call <vilib>:"Draw Flattened Pixmap.vi"("image data"=w222) -> ("new picture"=w211:picture)  [unwired: 8 in]
                    n111 = call <vilib>:"Draw Flattened Pixmap.vi"("image data"=w202) -> ("new picture"=w196:picture)  [unwired: 8 in]
                    n112 = property on="Robot Pose 1" class="XYGraph (strict)"("PlotImages.Back"=w211) -> ()  [unwired: 2 in, 2 out]
                    n113 = property on="Robot Pose 2" class="XYGraph (strict)"("PlotImages.Back"=w196) -> ()  [unwired: 2 in, 2 out]
                  }
                  frame Error {
                  }
                }
              }
            }
            n114 = case shown="True" w163 {
              frame False {
              }
              frame True {
                # "export the current robot pose data"
                n115 = Get Date/Time In Seconds() -> (seconds since 1Jan1904=w244:timestamp)
                n116 = Format Date/Time String(time format string (%c)="%Y-%m-%d_%H-%M", seconds (now)=w244) -> (date/time string=w242:string)  [unwired: 1 in]
                n117 = Concatenate Strings("robot pose data " ("string"), w242) -> (w240:string)
                n118 = Current VI's Path() -> (path=w239:path)
                n119 = String To Path(string=w240) -> (path=w236:path)
                n120 = Strip Path(path=w239) -> (stripped path=w238:path)  [unwired: 1 out]
                n121 = Strip Path(path=w238) -> (stripped path=w237:path)  [unwired: 1 out]
                n122 = Build Path(base path=w237, name or relative path=w236) -> (appended path=w235:path)
                n123 = invoke on="Robot Pose 1" class="XYGraph (strict)" method="Export Image"("FileType"=enum32{"BMP", "EPS", "EMF", "PICT"}."BMP" ("File Type"), "Target"=enum32{"File", "Clipboard"}."File", "Path"=w235, "HideGrid"=TRUE ("Hide Grid"), "Overwrite"=TRUE ("Always Overwrite")) -> ()  [unwired: 3 in, 8 out]
              }
            }
            n124 = property on="Robot Pose 2" class="XYGraph (strict)"("XScale.Maximum"=w123, "YScale.Maximum"=w124) -> ()  [unwired: 2 in, 2 out]
            n125 = call-poly <vilib>:"NT Read Value.vi"("default value"=0.0 ("Default Value"), "name"="Robot_P" ("Name")) -> ("value"=→"Robot_P":dbl)  [unwired: 7 in, 2 out]
            n126 = call-poly <vilib>:"NT Read Value.vi"("default value"=0.0 ("Default Value"), "name"="Robot_H" ("Name")) -> ("value"=w174:dbl)  [unwired: 7 in, 2 out]
            n127 = call-poly <vilib>:"NT Read Value.vi"("default value"=-1.0 ("Default Value"), "name"="Robot_Y" ("Name")) -> ("value"=w120:dbl)  [unwired: 7 in, 2 out]
            "Robot_Y" <- w120
            n128 = call-poly <vilib>:"NT Read Value.vi"("default value"=-1.0 ("Default Value"), "name"="Robot_X" ("Name")) -> ("value"=w119:dbl)  [unwired: 7 in, 2 out]
            "Robot_X" <- w119
            n129 = call-poly <vilib>:"NT Read Value.vi"("default value"=dbl[] [0.0, 0.0, 0.0, 0.0] ("Default Value"), "name"="Targeting_Information" ("Name")) -> ("value"=w121:dbl[])  [unwired: 7 in, 2 out]
            n130 = call-poly <vilib>:"NT Read Value.vi"("default value"=30.0 ("Default Value"), "name"="Robot_Width_Bumpers" ("Name")) -> ("value"=w143:dbl)  [unwired: 7 in, 2 out]
            n131 = call-poly <vilib>:"NT Read Value.vi"("default value"=30.0 ("Default Value"), "name"="Robot_Length_Bumpers" ("Name")) -> ("value"=w144:dbl)  [unwired: 7 in, 2 out]
            n132 = Quotient & Remainder(x=w174, y=360.0) -> (x-y*floor(x/y)=→"Robot_H_GUI":dbl)  [unwired: 1 out]
            n133 = call-poly <vilib>:"NT Read Value.vi"("default value"=w87, "name"="Auto_Path_Xs" ("Name")) -> ("value"=w88:dbl[])  [unwired: 7 in, 2 out]
            n134 = call-poly <vilib>:"NT Read Value.vi"("default value"=w87, "name"="Auto_Path_Ys" ("Name")) -> ("value"=w90:dbl[])  [unwired: 7 in, 2 out]
            n135 = Bundle("value"=w90, "value"=w88) -> (w92:cluster{"value":dbl[], "value":dbl[]})  [unwired: 1 in]
            n136 = call "RenderRobotPose.vi"("Robot X (in)"=w119, "Robot Width (in)"=w143, "Robot Length (in)"=w144, "Buffer Time (min)"=0.5, "Robot Y (in)"=w120, "Targeting Information"=w121, "Robot Heading (deg)"=w174, "Planned Path"=w92, "Robot Enabled"=TRUE, "Reset"="Clear_Robot_Pose_Display") -> ("Robot Pose"=→"Robot Pose 2" →"Robot Pose 1":cluster{dbl[], dbl[]}[])  [unwired: 5 in]
            n137 = local read "No_Secondary_Camera"() -> (w137:bool)
            n138 = property on="Robot Pose 2" class="XYGraph (strict)"("Visible"=w137) -> ()  [unwired: 2 in, 2 out]
            n139 = call-poly <vilib>:"NT Read Value.vi"("default value"=FALSE, "name"="Pointed_at_Target" ("Name")) -> ("value"=→"Pointed_at_Target":bool)  [unwired: 7 in, 2 out]
            n140 = call-poly <vilib>:"NT Read Value.vi"("name"="LL_Valid" ("Name")) -> ("value"=→"LL_Valid":bool)  [unwired: 8 in, 2 out]
            n141 = call-poly <vilib>:"NT Read Value.vi"("name"="Vision_Fault" ("Name")) -> ("value"=→"Vision_Fault_GUI":bool)  [unwired: 8 in, 2 out]
            n142 = call-poly <vilib>:"NT Read Value.vi"("default value"=0.0, "name"="Distance_to_Target" ("Name")) -> ("value"=→"Distance_to_Target":dbl)  [unwired: 7 in, 2 out]
            n143 = call-poly <vilib>:"NT Read Value.vi"("default value"=0.0, "name"="Heading_to_Target" ("Name")) -> ("value"=→"Heading_to_Target":dbl)  [unwired: 7 in, 2 out]
            n144 = call "ReducedBWSendToNT.vim"("Value In"="New_Blue_Calibration", "NT Name"="New_Blue_Calibration") -> ()  [unwired: 1 out]
            n145 = call-poly <vilib>:"NT Read Value.vi"("default value"=0.0, "name"="Current_Blue_Calibration" ("NT Name")) -> ("value"=w93:dbl)  [unwired: 7 in, 2 out]
            "Current_Blue_Calibration" <- w93
            n146 = call "ReducedBWSendToNT.vim"("Value In"="New_Red_Calibration", "NT Name"="New_Red_Calibration") -> ()  [unwired: 1 out]
            n147 = call "ReducedBWSendToNT.vim"("Value In"="Apply_Grid_Calibration", "NT Name"="Apply_Grid_Calibration") -> ()  [unwired: 1 out]
            n148 = call-poly <vilib>:"NT Read Value.vi"("default value"=0.0, "name"="Current_Red_Calibration" ("NT Name")) -> ("value"=w99:dbl)  [unwired: 7 in, 2 out]
            "Current_Red_Calibration" <- w99
            n149 = call "Is Value Changed.vim"("value"=w93) -> ("changed or first call?"=w94:bool)
            n150 = call "Is Value Changed.vim"("value"=w99) -> ("changed or first call?"=w100:bool)
            n151 = case shown="True" w94 {
              tunnel: w93 -> [_ w175]
              frame False {
              }
              frame True {
                n152 = property on="New_Blue_Calibration" class="DigNum (strict)"("Value"=w175) -> ()  [unwired: 2 in, 2 out]
              }
            }
            n153 = case shown="True" w100 {
              tunnel: w99 -> [_ w176]
              frame False {
              }
              frame True {
                n154 = property on="New_Red_Calibration" class="DigNum (strict)"("Value"=w176) -> ()  [unwired: 2 in, 2 out]
              }
            }
          }
          frame #2 {
            # "driver control configuration"
            # "robot configuration"
            # "robot and driver control configuration"
            n155 = local read "Dashboard Tab"() -> (w245:T1)
            n156 = case shown="\"Setup/Auto\"" w245 {
              frame "Checklist", Default {
              }
              frame "Setup/Auto" {
                n157 = call-poly <vilib>:"NT Read Value.vi"("default value"="No robot profile..." ("Default Value"), "name"="Robot_Profile" ("Name")) -> ("value"=→"Robot_Profile_GUI":string)  [unwired: 7 in, 2 out]
              }
            }
            n158 = Build Array("N/A") -> (w256:string[])
            n159 = And(x="Calibrate_Joysticks_GUI", y="Arm_Calibrate_Joysticks") -> (x .and. y?=w246:bool)
            n160 = To Double Precision Float(number="Select Driver Profile") -> (double precision float=w249:dbl)
            n161 = call-poly <vilib>:"NT Read Value.vi"("default value"=w256, "name"="Legal_Drivers" ("Name")) -> ("value"=w255:string[])  [unwired: 7 in, 2 out]
            "Legal_Drivers_GUI" <- w255
            n162 = Not(x="Arm_Calibrate_Joysticks") -> (.not. x?=w258:bool)
            n163 = call "ReducedBWSendToNT.vim"("Value In"=w249, "NT Name"="Selected_Driver" ("Name")) -> ()  [unwired: 1 out]
            n164 = property on="Select Driver Profile" class="Ring (strict)"("Strings []"=w255) -> ()  [unwired: 2 in, 2 out]
            n165 = call "ReducedBWSendToNT.vim"("Value In"=w246, "NT Name"="Calibrate_Joysticks" ("Name")) -> ()  [unwired: 1 out]
            n166 = Select(t=cluster{u32, u32}[] [{11776947, 16448250}, {16448250, 16448250}] ("Colors [4]"), s=w258, f=cluster{u32, u32}[] [{6618880, 16448250}, {16448250, 16448250}] ("Colors [4]")) -> (s? t:f=w259:cluster{u32, u32}[])
            n167 = property on="Calibrate_Joysticks_GUI" class="Bool"("Colors [4]"=w259) -> ()  [unwired: 2 in, 2 out]
          }
          frame #3 {
            # "configure auto play"
            # "set robot pose"
            # "autonomous configuration"
            n168 = call "ReducedBWSendToNT.vim"("Value In"="Manual_Start_X", "NT Name"="Manual_Start_X" ("Name")) -> ()  [unwired: 1 out]
            n169 = call "ReducedBWSendToNT.vim"("Value In"="Manual_Start_Y", "NT Name"="Manual_Start_Y" ("Name")) -> ()  [unwired: 1 out]
            n170 = call "ReducedBWSendToNT.vim"("Value In"="Manual_Start_H", "NT Name"="Manual_Start_H" ("Name")) -> ()  [unwired: 1 out]
            n171 = call "ReducedBWSendToNT.vim"("Value In"="Disable_Fusion_While_Autonomous", "NT Name"="Disable_Fusion_While_Autonomous" ("Name")) -> ()  [unwired: 1 out]
            n172 = call "ReducedBWSendToNT.vim"("Value In"="Disable_Fusion_While_Disabled", "NT Name"="Disable_Fusion_While_Disabled" ("Name")) -> ()  [unwired: 1 out]
            n173 = call "ReducedBWSendToNT.vim"("Value In"="Push_Robot_Start_GUI", "NT Name"="Push_Robot_Start" ("Name")) -> ()  [unwired: 1 out]
            n174 = local read "Dashboard Tab"() -> (w272:T1)
            n175 = To Double Precision Float(number="TeleOp Starting State") -> (double precision float=w265:dbl)
            n176 = To Double Precision Float(number="Scoring Position") -> (double precision float=w267:dbl)
            n177 = To Double Precision Float(number="Select Autonomous Play") -> (double precision float=w275:dbl)
            n178 = call "ReducedBWSendToNT.vim"("Value In"=w265, "NT Name"="TeleOp Starting State" ("Name")) -> ()  [unwired: 1 out]
            n179 = call "ReducedBWSendToNT.vim"("Value In"=w267, "NT Name"="Auto_Scoring_Position" ("Name")) -> ()  [unwired: 1 out]
            n180 = call "ReducedBWSendToNT.vim"("Value In"="Auto_Test_Mode_GUI", "NT Name"="Auto_Test_Mode" ("Name")) -> ()  [unwired: 1 out]
            n181 = call "ReducedBWSendToNT.vim"("Value In"="Auto_Delay_GUI", "NT Name"="Auto_Delay" ("Name")) -> ()  [unwired: 1 out]
            n182 = call "ReducedBWSendToNT.vim"("Value In"="Force_Human_Control_GUI", "NT Name"="Force_Human_Control" ("Name")) -> ()  [unwired: 1 out]
            n183 = call "ReducedBWSendToNT.vim"("Value In"=w275, "NT Name"="Selected_Auto_Play" ("Name")) -> ()  [unwired: 1 out]
            n184 = call "ReducedBWSendToNT.vim"("Value In"="Refresh_Auto_Play_List_GUI", "NT Name"="Refresh_Auto_Play_List" ("Name")) -> ()  [unwired: 1 out]
            n185 = case shown="\"Setup/Auto\"" w272 {
              tunnel: "Select Autonomous Play" -> [_ w295]
              tunnel: "Refresh_Auto_Play_List_GUI" -> [_ w294]
              frame "Checklist", Default {
              }
              frame "Setup/Auto" {
                w312 = "N/A" ("Default Value")
                n186 = call-poly <vilib>:"NT Read Value.vi"("default value"=0.0, "name"="Suggested_Start_H" ("Name")) -> ("value"=w311:dbl)  [unwired: 7 in, 2 out]
                n187 = call-poly <vilib>:"NT Read Value.vi"("default value"=0.0, "name"="Suggested_Start_X" ("Name")) -> ("value"=w309:dbl)  [unwired: 7 in, 2 out]
                n188 = call-poly <vilib>:"NT Read Value.vi"("default value"=0.0, "name"="Suggested_Start_Y" ("Name")) -> ("value"=w310:dbl)  [unwired: 7 in, 2 out]
                n189 = Build Array("N/A") -> (w315:string[])
                n190 = call "Is Value Changed.vim"("value"=w295) -> ("changed or first call?"=w296:bool)
                n191 = call "Is Value Changed.vim"("value"=w311) -> ("changed or first call?"=w302:bool)
                n192 = call "Is Value Changed.vim"("value"=w309) -> ("changed or first call?"=w298:bool)
                n193 = call "Is Value Changed.vim"("value"=w310) -> ("changed or first call?"=w300:bool)
                n194 = call-poly <vilib>:"NT Read Value.vi"("default value"=w312, "name"="Auto_Playbook" ("Name")) -> ("value"=→"Auto_Playbook_GUI":string)  [unwired: 7 in, 2 out]
                n195 = call-poly <vilib>:"NT Read Value.vi"("default value"=w312, "name"="Auto_Path_Suffix" ("Name")) -> ("value"=→"Auto_Suffix_GUI":string)  [unwired: 7 in, 2 out]
                n196 = call-poly <vilib>:"NT Read Value.vi"("default value"=w315, "name"="Legal_Auto_Plays" ("Name")) -> ("value"=w316:string[])  [unwired: 7 in, 2 out]
                n197 = Compound Arithmetic op=OR(w296, w294, w298) -> (w297:bool)
                n198 = Compound Arithmetic op=OR(w296, w294, w300) -> (w299:bool)
                n199 = Compound Arithmetic op=OR(w296, w294, w302) -> (w301:bool)
                n200 = property on="Select Autonomous Play" class="Ring (strict)"("Strings []"=w316) -> ()  [unwired: 2 in, 2 out]
                n201 = case shown="True" w301 {
                  tunnel: w311 -> [_ w321]
                  frame False {
                  }
                  frame True {
                    n202 = property on="Manual_Start_H" class="DigNum (strict)"("Value"=w321) -> ()  [unwired: 2 in, 2 out]
                  }
                }
                n203 = case shown="True" w299 {
                  tunnel: w310 -> [_ w322]
                  frame False {
                  }
                  frame True {
                    n204 = property on="Manual_Start_Y" class="DigNum (strict)"("Value"=w322) -> ()  [unwired: 2 in, 2 out]
                  }
                }
                n205 = case shown="True" w297 {
                  tunnel: w309 -> [_ w323]
                  frame False {
                  }
                  frame True {
                    n206 = property on="Manual_Start_X" class="DigNum (strict)"("Value"=w323) -> ()  [unwired: 2 in, 2 out]
                  }
                }
              }
            }
          }
          frame #4 {
            w344 = cluster{u32, u32}[] [{9567230, 16448250}, {16448250, 16448250}] ("Un-selected Color")
            w332 = bool[] [FALSE, FALSE] ("default value")
            w339 = bool[] [FALSE, FALSE, FALSE, FALSE, FALSE, FALSE] ("default value")
            w338 = bool[] [FALSE, FALSE, FALSE, FALSE, FALSE, FALSE] ("Default Value")
            w353 = cluster{u32, u32}[] [{9567230, 16448250}, {16448250, 16448250}] ("Un-selected Color")
            # "scoring states"
            # "master state controller"
            # "state indicators"
            n207 = global read "GlobalDashboard.vi" "Code_is_Running"() -> (w337:bool)
            n208 = call-poly <vilib>:"NT Read Value.vi"("default value"=w339, "name"="Confirmed_States" ("Name")) -> ("value"=w334:bool[])  [unwired: 7 in, 2 out]
            n209 = call-poly <vilib>:"NT Read Value.vi"("default value"=w338, "name"="Disallowed_States" ("Name")) -> ("value"=w336:bool[])  [unwired: 7 in, 2 out]
            n210 = Select(t=w336, s=w337, f=w338) -> (s? t:f=w335:bool[])
            n211 = Select(t=w334, s=w337, f=w339) -> (s? t:f=w333:bool[])
            n212 = Index Array(array=w335, index #1=0 ("index")) -> (element #1=w366:bool, element #2=w365:bool, element #3=w357:bool, element #4=w356:bool, element #5=w355:bool, element #6=w354:bool)  [unwired: 5 in]
            n213 = Index Array(array=w333, index #1=0 ("index")) -> (element #1=w372:bool, element #2=w368:bool, element #3=w328:bool, element #4=w326:bool, element #5=w358:bool, element #6=w327:bool)  [unwired: 5 in]
            "State_Shelf" <- w327
            "State_Score" <- w328
            "State_Hopper" <- w326
            n214 = call "ButtonColorChooser.vi"("Un-selected Color"=w353, "Disallowed"=w366, "Confirmed"=w372) -> ("Final Color"=w373:cluster{u32, u32}[])  [unwired: 8 in]
            n215 = call "ButtonColorChooser.vi"("Un-selected Color"=w353, "Disallowed"=w365, "Confirmed"=w368) -> ("Final Color"=w348:cluster{u32, u32}[])  [unwired: 8 in]
            n216 = call "ButtonColorChooser.vi"("Un-selected Color"=w353, "Disallowed"=w357, "Confirmed"=w328) -> ("Final Color"=w349:cluster{u32, u32}[])  [unwired: 8 in]
            n217 = call "ButtonColorChooser.vi"("Un-selected Color"=w353, "Disallowed"=w356, "Confirmed"=w326) -> ("Final Color"=w350:cluster{u32, u32}[])  [unwired: 8 in]
            n218 = call "ButtonColorChooser.vi"("Un-selected Color"=w353, "Disallowed"=w355, "Confirmed"=w358) -> ("Final Color"=w351:cluster{u32, u32}[])  [unwired: 8 in]
            n219 = call "ButtonColorChooser.vi"("Un-selected Color"=w353, "Disallowed"=w354, "Confirmed"=w327) -> ("Final Color"=w352:cluster{u32, u32}[])  [unwired: 8 in]
            n220 = property on="Master_State_STOW_Indicator" class="Bool (strict)"("Colors [4]"=w373) -> ()  [unwired: 2 in, 2 out]
            n221 = property on="Master_State_BLNC_Indicator" class="Bool (strict)"("Colors [4]"=w348) -> ()  [unwired: 2 in, 2 out]
            n222 = property on="Master_State_SCOR_Indicator" class="Bool (strict)"("Colors [4]"=w349) -> ()  [unwired: 2 in, 2 out]
            n223 = property on="Master_State_HOPR_Indicator" class="Bool (strict)"("Colors [4]"=w350) -> ()  [unwired: 2 in, 2 out]
            n224 = property on="Master_State_GRND_Indicator" class="Bool (strict)"("Colors [4]"=w351) -> ()  [unwired: 2 in, 2 out]
            n225 = property on="Master_State_SHLF_Indicator" class="Bool (strict)"("Colors [4]"=w352) -> ()  [unwired: 2 in, 2 out]
            n226 = local read "Grabbed_Gamepiece_Enum"() -> (w341:enum16{"CUBE", "CONE"})
            n227 = global read "GlobalDashboard.vi" "Code_is_Running"() -> (w331:bool)
            n228 = case shown="\"CONE\"" w341 {
              tunnel: [cluster{u32, u32}[] [{8388863, 16448250}, {16448250, 16448250}] ("Un-selected Color") cluster{u32, u32}[] [{16776960, 16448250}, {16448250, 16448250}] ("Un-selected Color")] -> w340
              frame "CUBE", Default {
              }
              frame "CONE" {
              }
            }
            n229 = call-poly <vilib>:"NT Read Value.vi"("default value"=w332, "name"="Confirmed_Score_States" ("Name")) -> ("value"=w330:bool[])  [unwired: 7 in, 2 out]
            n230 = Select(t=w330, s=w331, f=w332) -> (s? t:f=w329:bool[])
            n231 = Index Array(array=w329) -> (element #1=w346:bool, element #2=w345:bool)  [unwired: 2 in]
            n232 = Select(t=w340, s=w345, f=w344) -> (s? t:f=w324:cluster{u32, u32}[])
            n233 = Select(t=w340, s=w346, f=w344) -> (s? t:f=w325:cluster{u32, u32}[])
            n234 = property on="Score_State_LVL2_Indicator" class="Bool (strict)"("Colors [4]"=w324) -> ()  [unwired: 2 in, 2 out]
            n235 = property on="Score_State_LVL1_Indicator" class="Bool (strict)"("Colors [4]"=w325) -> ()  [unwired: 2 in, 2 out]
            "Master_State_STOW_Indicator" <- FALSE ("Master_State_0_Indicator")
            "Master_State_BLNC_Indicator" <- FALSE ("Master_State_0_Indicator")
            "Master_State_SCOR_Indicator" <- FALSE ("Master_State_0_Indicator")
            "Master_State_HOPR_Indicator" <- FALSE ("Master_State_0_Indicator")
            "Master_State_GRND_Indicator" <- FALSE ("Master_State_0_Indicator")
            "Master_State_SHLF_Indicator" <- FALSE ("Master_State_0_Indicator")
            "Score_State_LVL1_Indicator" <- FALSE ("Score_State_LVL1_Indicator")
            "Score_State_LVL2_Indicator" <- FALSE ("Score_State_LVL2_Indicator")
          }
          frame #5 {
            # "actuator test interlocks"
            # "emergency overrides"
            # "emergency overrides and interlocks"
            n236 = global read "GlobalDashboard.vi" "Code_is_Running"() -> (w379:bool)
            n237 = call-poly <vilib>:"NT Read Value.vi"("default value"=FALSE, "name"="Robot_in_Safety_Override" ("Name")) -> ("value"=w381:bool)  [unwired: 7 in, 2 out]
            n238 = call "EdgeTrigger.vi"("Input Signal"=w381) -> ("All Edge Trigger"=w382:bool)  [unwired: 2 out]
            n239 = call "EdgeTrigger.vi"("Input Signal"=w379) -> ("Falling Edge Trigger"=w378:bool)  [unwired: 2 out]
            n240 = call "ReducedBWSendToNT.vim"("Value In"="Clear_Errors_GUI", "NT Name"="Clear_Errors" ("Name")) -> ()  [unwired: 1 out]
            n241 = call "ReducedBWSendToNT.vim"("Value In"="Super_Test_Mode_GUI", "NT Name"="Super_Test_Mode" ("Name")) -> ()  [unwired: 1 out]
            n242 = call "ReducedBWSendToNT.vim"("Value In"="Auto_Targeting_Override", "NT Name"="Auto_Targeting_Override" ("Name")) -> ()  [unwired: 1 out]
            n243 = call "ReducedBWSendToNT.vim"("Value In"="Camera_Override_GUI", "NT Name"="Camera_Override" ("Name")) -> ()  [unwired: 1 out]
            n244 = call "ReducedBWSendToNT.vim"("Value In"="Field_Oriented_Override_GUI", "NT Name"="Field_Oriented_Override" ("Name")) -> ()  [unwired: 1 out]
            n245 = case shown="True" w382 {
              tunnel: w381 -> [_ w407]
              frame False {
              }
              frame True {
                n246 = property on="Master_Safety_Override_1" class="Bool (strict)"("Value"=w407) -> ()  [unwired: 2 in, 2 out]
              }
            }
            n247 = case shown="True" w378 {
              frame False {
              }
              frame True {
                n248 = property on="Master_Safety_Override_1" class="Bool (strict)"("Value"=FALSE ("Master_Safety_Override_1")) -> ()  [unwired: 2 in, 2 out]
              }
            }
            n249 = call "ReducedBWSendToNT.vim"("Value In"="Master_Safety_Override_1", "NT Name"="Master_Safety_Override" ("Name")) -> ()  [unwired: 1 out]
            n250 = property on="Actuator Testing" class="Ring (strict)"() -> ("RingText.Text"=w391:string)  [unwired: 2 in, 2 out]
            n251 = Build Array("No_Test") -> (w405:string[])
            n252 = call "ReducedBWSendToNT.vim"("Value In"="Free_Tuning_Variable_GUI", "NT Name"="Free_Tuning_Variable" ("Name")) -> ()  [unwired: 1 out]
            n253 = call-poly <vilib>:"NT Read Value.vi"("default value"=w405, "name"="Legal_Actuator_Names" ("Name")) -> ("value"=w404:string[])  [unwired: 7 in, 2 out]
            n254 = call "ReducedBWSendToNT.vim"("Value In"=w391, "NT Name"="Test_Actuator_Name" ("Name")) -> ()  [unwired: 1 out]
            n255 = call "ReducedBWSendToNT.vim"("Value In"="Test_Actuator_Value_GUI", "NT Name"="Test_Actuator_Value" ("Name")) -> ()  [unwired: 1 out]
            n256 = call "ReducedBWSendToNT.vim"("Value In"="Test_Actuator_Period_GUI", "NT Name"="Test_Actuator_Period" ("Name")) -> ()  [unwired: 1 out]
            n257 = property on="Actuator Testing" class="Ring (strict)"("Strings []"=w404) -> ()  [unwired: 2 in, 2 out]
          }
          frame #6 {
            # "drivebase subsytem"
            n258 = call "SwerveModuleReadData.vi"("NT Name (Errors)"="Swerve_1_Errors", "NT Name (Details)"="Swerve_1_Details" ("NT Name (Tune)")) -> ("Shifter State"=→"Swerve_1_Shifter_State":string, "Drive Velocity"=→"Swerve_1_Drive_Velocity":dbl, "Drive Temperature"=→"Swerve_1_Drive_Temperature":dbl, "Azimuth Position"=→"Swerve_1_Azimuth_Position":dbl, "Shifter Failure"=w474:T21, "Drive Overheating"=w476:T21, "Drive Fault"=w421:T21, "Azimuth Fault"=w475:T21)  [unwired: 2 in]
            n259 = call "SwerveModuleReadData.vi"("NT Name (Errors)"="Swerve_0_Errors", "NT Name (Details)"="Swerve_0_Details" ("NT Name (Tune)")) -> ("Shifter State"=→"Swerve_0_Shifter_State":string, "Drive Velocity"=→"Swerve_0_Drive_Velocity":dbl, "Drive Temperature"=→"Swerve_0_Drive_Temperature":dbl, "Azimuth Position"=→"Swerve_0_Azimuth_Position":dbl, "Shifter Failure"=w482:T21, "Drive Overheating"=w490:T21, "Drive Fault"=w423:T21, "Azimuth Fault"=w486:T21)  [unwired: 2 in]
            n260 = call-poly <vilib>:"NT Read Value.vi"("name"="Field_Oriented" ("Name")) -> ("value"=→"Field_Oriented_GUI":bool)  [unwired: 8 in, 2 out]
            n261 = call-poly <vilib>:"NT Read Value.vi"("name"="IMU_Failure" ("Name")) -> ("value"=→"IMU_Failure_GUI":bool)  [unwired: 8 in, 2 out]
            n262 = call "SwerveModuleReadData.vi"("NT Name (Errors)"="Swerve_2_Errors", "NT Name (Details)"="Swerve_2_Details" ("NT Name (Tune)")) -> ("Shifter State"=→"Swerve_2_Shifter_State":string, "Drive Velocity"=→"Swerve_2_Drive_Velocity":dbl, "Drive Temperature"=→"Swerve_2_Drive_Temperature":dbl, "Azimuth Position"=→"Swerve_2_Azimuth_Position":dbl, "Shifter Failure"=w469:T21, "Drive Overheating"=w471:T21, "Drive Fault"=w419:T21, "Azimuth Fault"=w470:T21)  [unwired: 2 in]
            n263 = call "SwerveModuleReadData.vi"("NT Name (Errors)"="Swerve_3_Errors", "NT Name (Details)"="Swerve_3_Details" ("NT Name (Tune)")) -> ("Shifter State"=→"Swerve_3_Shifter_State":string, "Drive Velocity"=→"Swerve_3_Drive_Velocity":dbl, "Drive Temperature"=→"Swerve_3_Drive_Temperature":dbl, "Azimuth Position"=→"Swerve_3_Azimuth_Position":dbl, "Shifter Failure"=w464:T21, "Drive Overheating"=w466:T21, "Drive Fault"=w417:T21, "Azimuth Fault"=w465:T21)  [unwired: 2 in]
            n264 = Unbundle(w476) -> ("Boolean"=w462:bool, "Numeric Text.Text Colors:Text Color"=w459:u32)
            n265 = Unbundle(w475) -> ("Boolean"=w463:bool, "Numeric Text.Text Colors:Text Color"=w460:u32)
            n266 = Unbundle(w490) -> ("Boolean"=w488:bool, "Numeric Text.Text Colors:Text Color"=w489:u32)
            n267 = Unbundle(w486) -> ("Boolean"=w485:bool, "Numeric Text.Text Colors:Text Color"=w483:u32)
            n268 = Unbundle(w474) -> ("Boolean"=w461:bool, "Numeric Text.Text Colors:Text Color"=w454:u32)
            n269 = Unbundle(w471) -> ("Boolean"=w452:bool, "Numeric Text.Text Colors:Text Color"=w450:u32)
            n270 = Unbundle(w482) -> ("Boolean"=w480:bool, "Numeric Text.Text Colors:Text Color"=w481:u32)
            n271 = Unbundle(w423) -> ("Boolean"=w415:bool, "Numeric Text.Text Colors:Text Color"=w424:u32)
            n272 = Unbundle(w470) -> ("Boolean"=w453:bool, "Numeric Text.Text Colors:Text Color"=w451:u32)
            n273 = Unbundle(w466) -> ("Boolean"=w441:bool, "Numeric Text.Text Colors:Text Color"=w440:u32)
            n274 = Unbundle(w465) -> ("Boolean"=w442:bool, "Numeric Text.Text Colors:Text Color"=w443:u32)
            n275 = Unbundle(w421) -> ("Boolean"=w414:bool, "Numeric Text.Text Colors:Text Color"=w422:u32)
            n276 = Unbundle(w469) -> ("Boolean"=w445:bool, "Numeric Text.Text Colors:Text Color"=w444:u32)
            n277 = Unbundle(w419) -> ("Boolean"=w413:bool, "Numeric Text.Text Colors:Text Color"=w420:u32)
            n278 = Unbundle(w464) -> ("Boolean"=w434:bool, "Numeric Text.Text Colors:Text Color"=w435:u32)
            n279 = Unbundle(w417) -> ("Boolean"=w412:bool, "Numeric Text.Text Colors:Text Color"=w418:u32)
            n280 = property on="Swerve_3_Drive_Velocity" class="DigNum (strict)"("NumText.BG Color"=w418) -> ()  [unwired: 2 in, 2 out]
            n281 = property on="Swerve_0_Azimuth_Position" class="DigNum (strict)"("NumText.BG Color"=w483) -> ()  [unwired: 2 in, 2 out]
            n282 = property on="Swerve_0_Drive_Temperature" class="DigNum (strict)"("NumText.BG Color"=w489) -> ()  [unwired: 2 in, 2 out]
            n283 = property on="Swerve_0_Shifter_State" class="Str"("Text.BG Color"=w481) -> ()  [unwired: 2 in, 2 out]
            n284 = property on="Swerve_1_Azimuth_Position" class="DigNum (strict)"("NumText.BG Color"=w460) -> ()  [unwired: 2 in, 2 out]
            n285 = property on="Swerve_1_Drive_Temperature" class="DigNum (strict)"("NumText.BG Color"=w459) -> ()  [unwired: 2 in, 2 out]
            n286 = property on="Swerve_1_Shifter_State" class="Str"("Text.BG Color"=w454) -> ()  [unwired: 2 in, 2 out]
            n287 = property on="Swerve_2_Azimuth_Position" class="DigNum (strict)"("NumText.BG Color"=w451) -> ()  [unwired: 2 in, 2 out]
            n288 = property on="Swerve_2_Drive_Temperature" class="DigNum (strict)"("NumText.BG Color"=w450) -> ()  [unwired: 2 in, 2 out]
            n289 = property on="Swerve_2_Shifter_State" class="Str"("Text.BG Color"=w444) -> ()  [unwired: 2 in, 2 out]
            n290 = property on="Swerve_3_Azimuth_Position" class="DigNum (strict)"("NumText.BG Color"=w443) -> ()  [unwired: 2 in, 2 out]
            n291 = property on="Swerve_3_Drive_Temperature" class="DigNum (strict)"("NumText.BG Color"=w440) -> ()  [unwired: 2 in, 2 out]
            n292 = property on="Swerve_3_Shifter_State" class="Str"("Text.BG Color"=w435) -> ()  [unwired: 2 in, 2 out]
            n293 = property on="Swerve_0_Drive_Velocity" class="DigNum (strict)"("NumText.BG Color"=w424) -> ()  [unwired: 2 in, 2 out]
            n294 = property on="Swerve_2_Drive_Velocity" class="DigNum (strict)"("NumText.BG Color"=w420) -> ()  [unwired: 2 in, 2 out]
            n295 = property on="Swerve_1_Drive_Velocity" class="DigNum (strict)"("NumText.BG Color"=w422) -> ()  [unwired: 2 in, 2 out]
            n296 = call-poly <vilib>:"NT Read Value.vi"("name"="Using_Auto_Targeting" ("Name")) -> ("value"=→"Using_Auto_Targeting":bool)  [unwired: 8 in, 2 out]
            n297 = Build Array(w480, w461, w445, w434) -> (→"Swerve_Shifter_Failure_Array":bool[])
            n298 = Build Array(w485, w463, w453, w442) -> (→"Swerve_Azimuth_Fault_Array":bool[])
            n299 = Build Array(w488, w462, w452, w441) -> (→"Swerve_Overheating_Array":bool[])
            n300 = Build Array(w415, w414, w413, w412) -> (→"Swerve_Drive_Fault_Array":bool[])
            n301 = local read "Dashboard Tab"() -> (w425:T1)
            n302 = case shown="\"Tune\"" w425 {
              frame "Checklist", Default {
              }
              frame "Tune" {
                n303 = call-poly <vilib>:"NT Read Value.vi"("default value"=dbl[] [0.0, 0.0, 0.0, 0.0, 0.0, 0.0] ("Default Value"), "name"="Current_Driver_Profile_Setpoints" ("Name")) -> ("value"=w515:dbl[])  [unwired: 7 in, 2 out]
                n304 = Array To Cluster(array=w515) -> (cluster=w511:T22)
                "Current_Driver_Profile_Setpoints_GUI" <- w511
                n305 = feedback #3(dbl[] [0.0, 0.0, 0.0, 0.0, 0.0, 0.0] ("Default Value")) -> (w514:dbl[])
                n306 = feedback-in #3(w515) -> ()
                n307 = Not Equal?(x=w515, y=w514) -> (x != y?=w513:bool[])
                n308 = Or Array Elements(Boolean array=w513) -> (logical OR=w512:bool)
                n309 = case shown="True" w512 {
                  tunnel: w511 -> [_ w519]
                  frame False {
                  }
                  frame True {
                    n310 = property on="New_Driver_Profile_Setpoints_GUI" class="Clust (strict)"("Value"=w519) -> ()  [unwired: 2 in, 2 out]
                  }
                }
              }
            }
            n311 = local read "Select Driver Profile"() -> (w499:u16)
            n312 = local read "Legal_Drivers_GUI"() -> (w500:string[])
            n313 = Cluster To Array(cluster="New_Driver_Profile_Setpoints_GUI") -> (array=w429:dbl[])
            n314 = And(x="Calibrate_Wheels_GUI", y="Arm_Calibrate_Wheels_GUI") -> (x .and. y?=w432:bool)
            n315 = Not(x="Arm_Calibrate_Wheels_GUI") -> (.not. x?=w506:bool)
            n316 = To Long Integer(number=w499) -> (32bit integer=w497:i32)
            n317 = call "ReducedBWSendToNT.vim"("Value In"="Home_Wheels_GUI", "NT Name"="Home_Wheels" ("Name")) -> ()  [unwired: 1 out]
            n318 = Index Array(array=w500, index=w497) -> (element=→"Current_Driver_Profile_GUI":string)
            n319 = call "ReducedBWSendToNT.vim"("Value In"="Apply_Driver_Profile_Setpoints_GUI", "NT Name"="Apply_Driver_Profile_Setpoints" ("Name")) -> ()  [unwired: 1 out]
            n320 = call "ReducedBWSendToNT.vim"("Value In"=w429, "NT Name"="New_Driver_Profile_Setpoints" ("Name")) -> ()  [unwired: 1 out]
            n321 = call "ReducedBWSendToNT.vim"("Value In"=w432, "NT Name"="Calibrate_Wheels" ("Name")) -> ()  [unwired: 1 out]
            n322 = call "ReducedBWSendToNT.vim"("Value In"="Arm_Calibrate_Wheels_GUI", "NT Name"="Unlock_Azimuth") -> ()  [unwired: 1 out]
            n323 = Select(t=cluster{u32, u32}[] [{11776947, 16448250}, {16448250, 16448250}] ("Colors [4]"), s=w506, f=cluster{u32, u32}[] [{6618880, 16448250}, {16448250, 16448250}] ("Colors [4]")) -> (s? t:f=w505:cluster{u32, u32}[])
            n324 = property on="Calibrate_Wheels_GUI" class="Bool"("Colors [4]"=w505) -> ()  [unwired: 2 in, 2 out]
          }
          frame #7 {
            w650 = dbl[] [0.0, 0.0, 0.0, 0.0] ("Default Value")
            w648 = dbl[] [0.0, 0.0, 0.0, 0.0] ("Default Value")
            # "get arm temperature\nmeasurements"
            # "arm and gripper subsystem"
            n325 = global read "GlobalDashboard.vi" "Code_is_Running"() -> (w558:bool)
            n326 = call-poly <vilib>:"NT Read Value.vi"("default value"=bool[] [FALSE, FALSE, FALSE], "name"="Arm_Motor_Over_Current") -> ("value"=w559:bool[])  [unwired: 7 in, 2 out]
            n327 = call-poly <vilib>:"NT Read Value.vi"("default value"=w648, "name"="Arm_Segment_Lengths") -> ("value"=w647:dbl[])  [unwired: 7 in, 2 out]
            n328 = call-poly <vilib>:"NT Read Value.vi"("default value"=w650, "name"="Arm_Base_Position") -> ("value"=w649:dbl[])  [unwired: 7 in, 2 out]
            n329 = call-poly <vilib>:"NT Read Value.vi"("default value"=bool[] [FALSE, FALSE, FALSE], "name"="Arm_Motor_Fault") -> ("value"=w565:bool[])  [unwired: 7 in, 2 out]
            n330 = call-poly <vilib>:"NT Read Value.vi"("default value"=bool[] [FALSE, FALSE, FALSE], "name"="Arm_Overheating") -> ("value"=w609:bool[])  [unwired: 7 in, 2 out]
            n331 = call-poly <vilib>:"NT Read Value.vi"("default value"=dbl[] [-1.0, -1.0, -1.0, 0.0] ("Default Value"), "name"="Arm_Temperatures") -> ("value"=w577:dbl[])  [unwired: 7 in, 2 out]
            n332 = Not Equal?(x=w650, y=w649) -> (x != y?=w645:bool[])
            n333 = Not Equal?(x=w648, y=w647) -> (x != y?=w646:bool[])
            n334 = Compound Arithmetic op=AND(w558, w559) -> (w555:bool[])
            "Arm_Motor_Over_Current_Array" <- w555
            n335 = call-poly <vilib>:"NT Read Value.vi"("default value"=FALSE, "name"="Gripper_Overheating") -> ("value"=w531:bool)  [unwired: 7 in, 2 out]
            "Gripper_Overheating" <- w531
            n336 = call-poly <vilib>:"NT Read Value.vi"("default value"=FALSE, "name"="Gripper_Motor_Fault") -> ("value"=w527:bool)  [unwired: 7 in, 2 out]
            "Gripper_Motor_Fault" <- w527
            n337 = Compound Arithmetic op=AND(w558, w565) -> (w557:bool[])
            "Arm_Motor_Fault_Array" <- w557
            n338 = Or Array Elements(Boolean array=w645) -> (logical OR=w644:bool)
            n339 = Or Array Elements(Boolean array=w646) -> (logical OR=w643:bool)
            n340 = Compound Arithmetic op=AND(w558, w609) -> (w586:bool[])
            "Arm_Overheating_Array" <- w586
            n341 = Index Array(array=w586) -> (element #1=w616:bool, element #2=w611:bool, element #3=w610:bool)  [unwired: 3 in]
            n342 = Or(x=w557, y=w555) -> (x .or. y?=w556:bool[])
            n343 = And(x=w644, y=w643) -> (x .and. y?=w642:bool)
            n344 = Index Array(array=w577) -> (element #1=→"Shoulder_Temp":dbl, element #2=→"Ebow_Temp":dbl, element #3=→"Wrist_Temp":dbl)  [unwired: 3 in]
            n345 = Index Array(array=w556) -> (element #1=w572:bool, element #2=w567:bool, element #3=w566:bool)  [unwired: 3 in]
            n346 = call "EdgeTrigger.vi"("Input Signal"=w642) -> ("Rising Edge Trigger"=w641:bool)  [unwired: 2 out]
            n347 = Select(t=u32 16711680 ("Numeric Text.Text Colors:Text Color"), s=w531, f=u32 4934475 ("Numeric Text.Text Colors:Text Color")) -> (s? t:f=w532:u32)
            n348 = Select(t=u32 16711680 ("Numeric Text.Text Colors:Text Color"), s=w527, f=u32 4934475 ("Numeric Text.Text Colors:Text Color")) -> (s? t:f=w528:u32)
            n349 = property on="Gripper_Temperature" class="DigNum (strict)"("NumText.BG Color"=w532) -> ()  [unwired: 2 in, 2 out]
            n350 = property on="Gripper_Velocity" class="DigNum (strict)"("NumText.BG Color"=w528) -> ()  [unwired: 2 in, 2 out]
            n351 = Select(t=u32 16711680 ("Numeric Text.Text Colors:Text Color"), s=w616, f=u32 4934475 ("Numeric Text.Text Colors:Text Color")) -> (s? t:f=w608:u32)
            n352 = Select(t=u32 16711680 ("Numeric Text.Text Colors:Text Color"), s=w611, f=u32 4934475 ("Numeric Text.Text Colors:Text Color")) -> (s? t:f=w607:u32)
            n353 = Select(t=u32 16711680 ("Numeric Text.Text Colors:Text Color"), s=w610, f=u32 4934475 ("Numeric Text.Text Colors:Text Color")) -> (s? t:f=w606:u32)
            n354 = Select(t=u32 16711680 ("Numeric Text.Text Colors:Text Color"), s=w572, f=u32 4934475 ("Numeric Text.Text Colors:Text Color")) -> (s? t:f=w564:u32)
            n355 = Select(t=u32 16711680 ("Numeric Text.Text Colors:Text Color"), s=w567, f=u32 4934475 ("Numeric Text.Text Colors:Text Color")) -> (s? t:f=w563:u32)
            n356 = Select(t=u32 16711680 ("Numeric Text.Text Colors:Text Color"), s=w566, f=u32 4934475 ("Numeric Text.Text Colors:Text Color")) -> (s? t:f=w562:u32)
            n357 = property on="Shoulder_Temp" class="DigNum (strict)"("NumText.BG Color"=w608) -> ()  [unwired: 2 in, 2 out]
            n358 = property on="Ebow_Temp" class="DigNum (strict)"("NumText.BG Color"=w607) -> ()  [unwired: 2 in, 2 out]
            n359 = property on="Wrist_Temp" class="DigNum (strict)"("NumText.BG Color"=w606) -> ()  [unwired: 2 in, 2 out]
            n360 = property on="Shoulder_Current_Angle" class="DigNum (strict)"("NumText.BG Color"=w564) -> ()  [unwired: 2 in, 2 out]
            n361 = property on="Ebow_Current_Angle" class="DigNum (strict)"("NumText.BG Color"=w563) -> ()  [unwired: 2 in, 2 out]
            n362 = property on="Wrist_Current_Angle" class="DigNum (strict)"("NumText.BG Color"=w562) -> ()  [unwired: 2 in, 2 out]
            n363 = feedback #4() -> (w654:errorcluster)  [unwired: 1 in]
            n364 = feedback #5() -> (w653:refnum<class "NI_Robotics_Serial Robot Arm.lvclass">)  [unwired: 1 in]
            n365 = feedback #6(FALSE) -> (w652:bool)
            n366 = case shown="True" w641 {
              tunnel: [w717 w723] -> w633
              tunnel: [w718 w722] -> w631
              tunnel: w647 -> [_ w734]
              tunnel: w649 -> [_ w725]
              tunnel: w654 -> [w718 _]
              tunnel: w653 -> [w717 _]
              tunnel: [w716 w719] -> w626
              tunnel: w652 -> [w716 _]
              frame False {
              }
              frame True {
                w724 = T23 {"twist angle"=0.0, "length"=0.0, "rotation angle"=0.0, "offset distance"=0.0, "joint type"=enum."Revolute", "joint coordinate offset"=0.0} ("Link Parameters")
                # "define the serial arm parameters"
                n367 = Index Array(array=w734) -> (element #1=w733:dbl, element #2=w732:dbl, element #3=w731:dbl)  [unwired: 3 in]
                n368 = expression code="(x/180.0)*pi" ("degrees to radians")(90.0 ("twist angle")) -> (w741:dbl)
                n369 = expression code="x*0.0254" ("degrees to radians")(w732) -> (w743:dbl)
                n370 = expression code="x*0.0254" ("degrees to radians")(w733) -> (w744:dbl)
                n371 = expression code="x*0.0254" ("degrees to radians")(w731) -> (w742:dbl)
                n372 = Bundle By Name(cluster=w724, "twist angle"=w741) -> (w739:T23)
                n373 = Bundle By Name(cluster=w724, "length"=w744) -> (w738:T23)
                n374 = Bundle By Name(cluster=w724, "length"=w743) -> (w737:T23)
                n375 = Bundle By Name(cluster=w724, "length"=w742) -> (w736:T23)
                n376 = expression code="(x/180.0)*pi" ("degrees to radians")(cluster{"roll":dbl, "pitch":dbl, "yaw":dbl} {"roll"=0.0, "pitch"=0.0, "yaw"=180.0} ("angles")) -> (w728:cluster{"roll":dbl, "pitch":dbl, "yaw":dbl})
                n377 = expression code="x*0.0254" ("degrees to radians")(w725) -> (w727:dbl[])
                n378 = Build Array(w739, w738, w737, w736) -> (w735:T23[])
                n379 = call <vilib>:"Roll Pitch Yaw to Rotation Matrix.vi"("angles"=w728) -> ("rotation matrix"=w730:T25)
                n380 = call <vilib>:"Rotation Matrix to Transform.vi"("translation vector"=w727, "rotation matrix"=w730) -> ("transform"=w726:T25)
                n381 = call-poly <vilib>:"Initialize Serial Arm.vi"("kinematic parameters"=w735) -> ("error out"=w745:errorcluster, "serial arm out"=w746:refnum<class "NI_Robotics_Serial Robot Arm.lvclass">)  [unwired: 9 in]
                n382 = call <vilib>:"Set Base Transform.vi"("error in (no error)"=w745, "base transform"=w726, "serial arm in"=w746) -> ("error out"=w722:errorcluster, "serial arm out"=w723:refnum<class "NI_Robotics_Serial Robot Arm.lvclass">)  [unwired: 7 in]
                n383 = Unbundle By Name(w722) -> ("status"=w721:bool)
                n384 = Or(x=w721, y=TRUE) -> (x .or. y?=w719:bool)
              }
            }
            n385 = feedback-in #4(w631) -> ()
            n386 = feedback-in #5(w633) -> ()
            n387 = feedback-in #6(w626) -> ()
            n388 = call-poly <vilib>:"NT Read Value.vi"("default value"=FALSE, "name"="Arm_Has_Arrived") -> ("value"=→"Arm_Has_Arrived":bool)  [unwired: 7 in, 2 out]
            n389 = call-poly <vilib>:"NT Read Value.vi"("default value"=0.0, "name"="Selected_Gamepiece") -> ("value"=w547:dbl)  [unwired: 7 in, 2 out]
            n390 = call-poly <vilib>:"NT Read Value.vi"("default value"=0.0, "name"="End_Effector_X") -> ("value"=→"End_Effector_X":dbl)  [unwired: 7 in, 2 out]
            n391 = call-poly <vilib>:"NT Read Value.vi"("default value"=0.0, "name"="End_Effector_Z") -> ("value"=→"End_Effector_Z":dbl)  [unwired: 7 in, 2 out]
            n392 = call-poly <vilib>:"NT Read Value.vi"("default value"=FALSE, "name"="Gamepiece_Grabbed") -> ("value"=→"Gamepiece_Grabbed_2" →"Gamepiece_Grabbed_1":bool)  [unwired: 7 in, 2 out]
            n393 = call-poly <vilib>:"NT Read Value.vi"("default value"=0.0, "name"="Gripper_Temperature") -> ("value"=→"Gripper_Temperature":dbl)  [unwired: 7 in, 2 out]
            n394 = call-poly <vilib>:"NT Read Value.vi"("default value"=0.0, "name"="Gripper_Velocity") -> ("value"=→"Gripper_Velocity":dbl)  [unwired: 7 in, 2 out]
            n395 = call "ReducedBWSendToNT.vim"("Value In"="Arm_Override", "NT Name"="Arm_Override" ("Name")) -> ()  [unwired: 1 out]
            n396 = call "ReducedBWSendToNT.vim"("Value In"="Jog Z (in)", "NT Name"="Jog_Z" ("Name")) -> ()  [unwired: 1 out]
            n397 = call "ReducedBWSendToNT.vim"("Value In"="Jog X (in)", "NT Name"="Jog_X" ("Name")) -> ()  [unwired: 1 out]
            n398 = Coerce To Type(0:w547, 1:enum16{"CUBE", "CONE"}."CUBE" ("Grabbed_Gamepiece")) -> (2:→"Grabbed_Gamepiece_Enum":enum16{"CUBE", "CONE"})
            n399 = First Call?() -> (First Call?: T/F=w638:bool)
            n400 = Or(x="Reset 3D View", y=w638) -> (x .or. y?=w637:bool)
            n401 = local read "Dashboard Tab"() -> (w628:T1)
            n402 = case shown="True" w637 {
              tunnel: T13 {"X"=0.0, "Y"=0.0, "Z"=1.0} ("Up Direction") -> [_ w663]
              tunnel: T13 {"X"=0.0, "Y"=0.0, "Z"=1.0} ("Target") -> [_ w662]
              tunnel: T13 {"X"=0.0, "Y"=3.35, "Z"=1.0} ("Camera Position") -> [_ w661]
              tunnel: w626 -> [w657 w660]
              tunnel: [w657 w660] -> w625
              tunnel: w633 -> [w656 w659]
              tunnel: [w656 w659] -> w632
              tunnel: w631 -> [w655 w658]
              tunnel: [w655 w658] -> w630
              frame False {
              }
              frame True {
                # "reset the camera view"
                n403 = invoke on="3D Arm Model" class="SceneGraphDisp (strict)" method="Setup Camera"("Camera Position"=w661, "Target"=w662, "Up Direction"=w663) -> ()  [unwired: 3 in, 6 out]
              }
            }
            n404 = Equal?(x=w628, y=T1."Tune") -> (x = y?=w623:bool)
            n405 = And(x=w623, y=w625) -> (x .and. y?=w624:bool)
            n406 = And(x="Calibrate_Arm", y="Arm_Calibrate_Arm") -> (x .and. y?=w593:bool)
            n407 = case shown="True" w624 {
              tunnel: w630 -> [_ w687]
              tunnel: w632 -> [_ w686]
              frame False {
              }
              frame True {
                # "render the 3D model"
                n408 = call-poly <vilib>:"NT Read Value.vi"("default value"=dbl[] [0.0, 0.0, 0.0, 0.0] ("Default Value"), "name"="Arm_Gripper_Goal") -> ("value"=w674:dbl[])  [unwired: 7 in, 2 out]
                n409 = call-poly <vilib>:"NT Read Value.vi"("default value"=dbl[] [0.0, 0.0, 0.0, 0.0] ("Default Value"), "name"="Arm_Current_Angles") -> ("value"=w668:dbl[])  [unwired: 7 in, 2 out]
                n410 = call "Is Value Changed.vim"("value"=w674) -> ("changed or first call?"=w672:bool)
                n411 = call "Is Value Changed.vim"("value"=w668) -> ("changed or first call?"=w673:bool)
                n412 = Build Array (concatenate)(0.0, w668) -> (w669:dbl[])
                n413 = Index Array(array=w668) -> (element #1=→"Shoulder_Current_Angle":dbl, element #2=→"Ebow_Current_Angle":dbl, element #3=→"Wrist_Current_Angle":dbl)  [unwired: 3 in]
                n414 = Compound Arithmetic op=OR(w673, w672) -> (w671:bool)
                n415 = expression code="(x/180.0)*pi" ("degrees to radians")(w669) -> (w676:dbl[])
                n416 = Index Array(array=w674) -> (element #1=w682:dbl, element #2=w681:dbl, element #3=w680:dbl)  [unwired: 3 in]
                n417 = call <vilib>:"Create Sphere.vi"("Color"=T14 {"Red"=0.0, "Green"=1.0, "Blue"=0.0, "Alpha"=1.0}, "Radius"=sgl 0.05) -> ("error out"=w688:errorcluster, "New Sphere Refnum"=w689:refnum<vi>)  [unwired: 8 in]
                n418 = Bundle("Numeric"=w682, "Numeric"=w681, "Numeric"=w680) -> (w679:T26)  [unwired: 1 in]
                n419 = expression code="x*0.0254" ("degrees to radians")(w679) -> (w683:T26)
                n420 = call <vilib>:"Create 3D Axis.vi"("Character Size"=sgl 0.2, "Axis label?"=TRUE, "Color"=T14 {"Red"=0.0, "Green"=1.0, "Blue"=1.0, "Alpha"=1.0}, "Radius"=sgl 0.01, "Length"=sgl 0.2, "Name"="XYZ axis") -> ("New Object Refnum"=w696:refnum<vi>)  [unwired: 4 in, 1 out]
                n421 = call-poly <vilib>:"Create Object.vi"("error in (no error)"=w688, "Geometry"=w689, "Name"="goal") -> ("error out"=w694:errorcluster, "Scene:New Object"=w692:refnum<vi>)  [unwired: 7 in]
                n422 = call <vilib>:"Set Translation.vi"("error in (no error)"=w694, "Translation"=w683, "Scene Object"=w692) -> ("Translated Object"=w695:refnum<vi>)  [unwired: 7 in, 1 out]
                n423 = feedback #7() -> (w670:refnum<vi>)  [unwired: 1 in]
                n424 = case shown="False" w671 {
                  tunnel: w696 -> [_ w714]
                  tunnel: w695 -> [_ w712]
                  tunnel: w687 -> [_ w707]
                  tunnel: w686 -> [_ w706]
                  tunnel: [w703 w705] -> w664
                  tunnel: w676 -> [_ w704]
                  tunnel: w670 -> [w703 _]
                  frame False {
                  }
                  frame True {
                    n425 = call <vilib>:"Initialize Plot.vi"("error in (no error)"=w707, "serial arm in"=w706) -> ("error out"=w708:errorcluster, "serial arm out"=w709:refnum<class "NI_Robotics_Serial Robot Arm.lvclass">)  [unwired: 8 in]
                    n426 = call <vilib>:"Update Plot.vi"("error in (no error)"=w708, "joint positions"=w704, "serial arm in"=w709) -> ("error out"=w711:errorcluster, "serial arm scene"=w715:refnum<vi>)  [unwired: 6 in, 1 out]
                    n427 = call-poly <vilib>:"Add Object.vi"("error in (no error)"=w711, "New Object In"=w714, "Scene Object In"=w715) -> ("error out"=w710:errorcluster, "Scene Object Out"=w713:refnum<vi>)  [unwired: 7 in]
                    n428 = call-poly <vilib>:"Add Object.vi"("error in (no error)"=w710, "New Object In"=w712, "Scene Object In"=w713) -> ("Scene Object Out"=w705:refnum<vi>)  [unwired: 7 in, 1 out]
                  }
                }
                "3D Arm Model" <- w664
                n429 = feedback-in #7(w664) -> ()
              }
            }
            n430 = call-poly <vilib>:"NT Read Value.vi"("default value"=FALSE, "name"="Gripper_Intaking") -> ("value"=→"Gripper_Intaking":bool)  [unwired: 7 in, 2 out]
            n431 = call-poly <vilib>:"NT Read Value.vi"("default value"=FALSE, "name"="Gripper_Outtaking") -> ("value"=→"Gripper_Outtaking":bool)  [unwired: 7 in, 2 out]
            n432 = Not(x="Arm_Calibrate_Arm") -> (.not. x?=w598:bool)
            n433 = call "ReducedBWSendToNT.vim"("Value In"="Simulate_Arm", "NT Name"="Simulate_Arm" ("Name")) -> ()  [unwired: 1 out]
            n434 = call "ReducedBWSendToNT.vim"("Value In"="Unlock_Arm_Joints", "NT Name"="Unlock_Arm_Joints" ("Name")) -> ()  [unwired: 1 out]
            n435 = call "ReducedBWSendToNT.vim"("Value In"=w593, "NT Name"="Calibrate_Arm" ("Name")) -> ()  [unwired: 1 out]
            n436 = Select(t=cluster{u32, u32}[] [{11776947, 16448250}, {16448250, 16448250}] ("Colors [4]"), s=w598, f=cluster{u32, u32}[] [{6618880, 16448250}, {16448250, 16448250}] ("Colors [4]")) -> (s? t:f=w599:cluster{u32, u32}[])
            n437 = property on="Calibrate_Arm" class="Bool"("Colors [4]"=w599) -> ()  [unwired: 2 in, 2 out]
          }
          frame #8 {
            # "intake subsystem"
          }
          frame #9 {
            w750 = bool[] [FALSE, FALSE, FALSE, FALSE, FALSE, FALSE, FALSE, FALSE, FALSE] ("Hybrid_Node_States")
            # "hybrid node indicators"
            # "combine errors for in-match reporting"
            # "manage targeting reticules"
            # "manage audible warnings"
            # "error management and driver assistance"
            n438 = local read "Arm_Motor_Over_Current_Array"() -> (w767:bool[])
            n439 = local read "Swerve_Azimuth_Fault_Array"() -> (w794:bool[])
            n440 = local read "Swerve_Shifter_Failure_Array"() -> (w797:bool[])
            n441 = local read "Swerve_Overheating_Array"() -> (w795:bool[])
            n442 = local read "Swerve_Drive_Fault_Array"() -> (w766:bool[])
            n443 = local read "Arm_Overheating_Array"() -> (w774:bool[])
            n444 = local read "Arm_Motor_Fault_Array"() -> (w768:bool[])
            n445 = Or Array Elements(Boolean array=w794) -> (logical OR=→"Swerve_Azimuth_Fault":bool)
            n446 = Or Array Elements(Boolean array=w795) -> (logical OR=→"Swerve_Overheating":bool)
            n447 = Or Array Elements(Boolean array=w797) -> (logical OR=→"Swerve_Shifter_Failure":bool)
            n448 = Or Array Elements(Boolean array=w766) -> (logical OR=→"Swerve_Drive_Fault":bool)
            n449 = Or Array Elements(Boolean array=w774) -> (logical OR=→"Arm_Overheating":bool)
            n450 = Or Array Elements(Boolean array=w768) -> (logical OR=→"Arm_Motor_Fault":bool)
            n451 = Or Array Elements(Boolean array=w767) -> (logical OR=→"Arm_Motor_Over_Current":bool)
            n452 = Build Array("Driver_Help", "Manipulator_Help") -> (w802:bool[])
            n453 = Or Array Elements(Boolean array=w802) -> (logical OR=w793:bool)
            n454 = Not(x=w793) -> (.not. x?=w810:bool)
            n455 = Build Array (concatenate)(w810, w802) -> (w809:bool[])
            n456 = property on="Help Graphic" class="ImageControl"("Visible"=w793) -> ()  [unwired: 2 in, 2 out]
            n457 = call "StateSelection.vi"("Disallowed States"=bool[] [FALSE, FALSE, FALSE, FALSE], "State Triggers"=w809, "State Names"=string[] ["No Help", "Driver Help", "Manipulator Help"]) -> ("Selected State"=w814:string)
            n458 = case shown="\"Driver Help\"" w814 {
              tunnel: [_ w835 w837] -> w796
              tunnel: w793 -> [_ _ _]
              frame "No Help", Default {
              }
              frame "Driver Help" {
                n459 = call "RenderJoystickDiagram.vi"("Joystick Graphic Filename"="driver joystick diagram.png") -> ("Image Out"=w835:T3)  [unwired: 10 in]
              }
              frame "Manipulator Help" {
                n460 = call "RenderJoystickDiagram.vi"("Joystick Graphic Filename"="manipulator joystick diagram.png") -> ("Image Out"=w837:T3)  [unwired: 10 in]
              }
            }
            "Help Graphic" <- w796
            n461 = Or Array Elements(Boolean array=w802) -> (logical OR=w804:bool)
            n462 = Not(x=w804) -> (.not. x?=w803:bool)
            n463 = Or(x=w803, y=w802) -> (x .or. y?=w801:bool[])
            n464 = Index Array(array=w801) -> (element #1=w773:bool, element #2=w772:bool)  [unwired: 2 in]
            n465 = Select(t=T15."Enabled" ("Disabled"), s=w772, f=T15."Disabled and Grayed Out" ("Disabled")) -> (s? t:f=w805:T15)
            n466 = Select(t=T15."Enabled" ("Disabled"), s=w773, f=T15."Disabled and Grayed Out" ("Disabled")) -> (s? t:f=w834:T15)
            n467 = property on="Driver_Help" class="Bool (strict)"("DisabledEnum"=w834) -> ()  [unwired: 2 in, 2 out]
            n468 = property on="Manipulator_Help" class="Bool (strict)"("DisabledEnum"=w805) -> ()  [unwired: 2 in, 2 out]
            n469 = call-poly <vilib>:"NT Read Value.vi"("name"="Alliance_Color" ("Name")) -> ("value"=w756:dbl)  [unwired: 8 in, 2 out]
            n470 = To Unsigned Word Integer(number=w756) -> (unsigned 16bit integer=w755:u16)
            n471 = call-poly <vilib>:"NT Read Value.vi"("default value"=0.0, "name"="Nearest_Hybrid_Node") -> ("value"=w751:dbl)  [unwired: 7 in, 2 out]
            n472 = Equal?(x=WPI_DriverStationAllianceInfo."Red", y=w755) -> (x = y?=→"Hybrid_Node_Names":bool)
            n473 = call-poly <vilib>:"NT Read Value.vi"("default value"=w750, "name"="Scored_Hybrid_Nodes") -> ("value"=→"Scored_Hybrid_Nodes":bool[])  [unwired: 7 in, 2 out]
            n474 = First Call?() -> (First Call?: T/F=w782:bool)
            n475 = To Long Integer(number=w751) -> (32bit integer=w752:i32)
            n476 = call-poly <vilib>:"NT Read Value.vi"("default value"=FALSE ("Default Value"), "name"="Master_Alarm" ("Name")) -> ("value"=w778:bool)  [unwired: 7 in, 2 out]
            n477 = call "Timer.vi"("Reset Timer"=w782) -> ("Time (ms)"=w781:u32)
            n478 = Insert Into Array(array=w750, index=w752, new element=TRUE ("new element/subarray")) -> (→"Nearest_Hybrid_Node":bool[])
            n479 = Greater?(x=w781, y=u32 2500) -> (0:w779:bool)
            n480 = local read "Arm_Calibrate_Wheels_GUI"() -> (w784:bool)
            n481 = call-poly <vilib>:"NT Read Value.vi"("default value"=0.0 ("Default Value"), "name"="Number_of_Master_Alarms" ("Name")) -> ("value"=w788:dbl)  [unwired: 7 in, 2 out]
            n482 = And(x=w779, y=w778) -> (x .and. y?=w777:bool)
            n483 = call "EdgeTrigger.vi"("Input Signal"="Mute_Audible_Warnings") -> ("Rising Edge Trigger"=w822:bool)  [unwired: 2 out]
            n484 = local read "Arm_Calibrate_Joysticks"() -> (w785:bool)
            n485 = To Long Integer(number=w788) -> (32bit integer=w787:i32)
            n486 = local read "Arm_Calibrate_Arm"() -> (w771:bool)
            n487 = call "BlinkLight.vi"() -> ("Blinked"=w827:bool)  [unwired: 1 in]
            n488 = Number To Decimal String(number=w787) -> (decimal integer string=w828:string)  [unwired: 1 in]
            n489 = feedback #8(TRUE ("t")) -> (w820:bool)
            n490 = Not(x=w820) -> (.not. x?=w819:bool)
            n491 = Select(t=w819, s=w822, f=w820) -> (s? t:f=w776:bool)
            "Audible_Warnings_Enabled_GUI" <- w776
            n492 = feedback-in #8(w776) -> ()
            n493 = Select(t=w827, s=w777, f=FALSE) -> (s? t:f=w831:bool)
            "Master_Caution_GUI_1" <- w831
            "Master_Caution_GUI_0" <- w831
            "Master_Caution_GUI_2" <- w831
            n494 = Concatenate Strings("MASTER ALARM (" ("string"), w828, ")" ("string")) -> (w829:string)
            n495 = Select(t=w829, s=w831, f="") -> (s? t:f=w830:string)
            n496 = Compound Arithmetic op=OR(w785, w784, w771) -> (w783:bool)
            n497 = local read "State_Hopper"() -> (→"WA_Ret_Left" →"WA_Ret_Right":bool)
            n498 = Select(t=cluster{u32, u32}[] [{6618880, 16448250}, {16448250, 16448250}] ("Colors [4]"), s=w776, f=cluster{u32, u32}[] [{16755474, 16448250}, {16448250, 16448250}] ("Colors [4]")) -> (s? t:f=w818:cluster{u32, u32}[])
            n499 = local read "State_Score"() -> (w763:bool)
            n500 = local read "State_Shelf"() -> (w762:bool)
            n501 = call "ReducedBWSendToNT.vim"("Value In"=w783, "NT Name"="Some_Switch_Armed" ("Name")) -> ()  [unwired: 1 out]
            n502 = property on="Master_Caution_GUI_0" class="Bool (strict)"("BoolText.Text"=w830) -> ()  [unwired: 2 in, 2 out]
            n503 = property on="Master_Caution_GUI_1" class="Bool (strict)"("BoolText.Text"=w830) -> ()  [unwired: 2 in, 2 out]
            n504 = property on="Master_Caution_GUI_2" class="Bool (strict)"("BoolText.Text"=w830) -> ()  [unwired: 2 in, 2 out]
            n505 = property on="Mute_Audible_Warnings" class="Bool"("Colors [4]"=w818) -> ()  [unwired: 2 in, 2 out]
            n506 = Or(x=w763, y=w762) -> (x .or. y?=→"LL_Ret_Left" →"LL_Ret_Right":bool)
          }
          frame #10 {
            # "flush NT tables"
            n507 = call <vilib>:"NT Flush Data Updates.vi"() -> ()  [unwired: 11 in, 1 out]
          }
        }
      }
    }
  }
  n508 = while {
    stop <- FALSE stop-if-true
    # "Set window properties"
    n509 = Not(x="Dock_Dashboard") -> (.not. x?=w840:bool)
    n510 = First Call?() -> (First Call?: T/F=w844:bool)
    n511 = Wait (ms)(milliseconds to wait=u32 10) -> ()  [unwired: 1 out]
    n512 = Compound Arithmetic op=OR(w840, w844) -> (w842:bool)
    n513 = control-ref of="This VI"() -> (w843:refnum<vi>)
    n514 = call "EdgeTrigger.vi"("Input Signal"=w842) -> ("Falling Edge Trigger"=w841:bool)  [unwired: 2 out]
    n515 = case shown="False" w842 {
      tunnel: w843 -> [w849 w856]
      tunnel: w841 -> [w847 _]
      frame False {
        n516 = case shown="True" w847 {
          tunnel: T27 {"Left"=100, "Top"=100, "Right"=1390, "Bottom"=585} ("Front Panel Window:Window Bounds") -> [_ w855]
          tunnel: w849 -> [w852 w854]
          tunnel: [w852 w853] -> w848
          frame False {
          }
          frame True {
            n517 = property class="VI"(reference=w854, "Front Panel.WinBounds"=w855) -> (reference out=w853:refnum<vi>)  [unwired: 1 in, 1 out]
          }
        }
        n518 = property class="VI"(reference=w848, "Front Panel.TitleBarVis"=TRUE ("Front Panel Window:Title Bar Visible")) -> ()  [unwired: 1 in, 2 out]
      }
      frame True {
        n519 = property class="VI"(reference=w856, "Front Panel.WinBounds"=T27 {"Left"=0, "Top"=0, "Right"=1290, "Bottom"=485} ("Front Panel Window:Window Bounds"), "Front Panel.TitleBarVis"=FALSE ("Front Panel Window:Title Bar Visible")) -> ()  [unwired: 1 in, 2 out]
      }
    }
  }
  n520 = while {
    tunnel: w20 -> [w862]
    tunnel: w19 -> [_]
    tunnel: w17 -> [w861]
    tunnel: w12 -> [w860]
    tunnel: w2 -> [w859]
    stop <- FALSE stop-if-true
    # "Process UI events related to test mode, checklist, and camera settings"
    n521 = event shown="[0] Timeout" {
      selector: w862 -> [_ _ _ _]
      dyn-events: _ -> [_ _ _ _]
      timeout: u32 60 ("milliseconds to wait") -> [_ _ _ _]
      tunnel: w861 -> [_ _ _ _]
      tunnel: w860 -> [_ _ _ _]
      tunnel: w859 -> [w865 _ _ _]
      event Timeout {
        (unwired) T1."Variables" ("Dashboard Tab")
        n522 = event-data() -> ()  [unwired: 1 in, 1 out]
        n523 = case shown="\"Variables\"" "Dashboard Tab" {
          tunnel: w865 -> [_ _ _]
          frame "Tune" {
          }
          frame "TeleOp", Default {
          }
          frame "Variables" {
            w870 = string[] ["CameraPublisher", "Usage", "DB"]  # Items to initially close
            n524 = First Call?() -> (First Call?: T/F=w871:bool)
            n525 = control-ref of="Tree"() -> (w872:refnum<vi>)
            n526 = Select(t=w870, s=w871, f=string[] []) -> (s? t:f=w868:string[])
            n527 = call <vilib>:"NT Read and Format Entries as Tree.vi"("Tags to  Close"=w868, "Tree Refnum"=w872) -> ()  [unwired: 8 in, 2 out]
          }
        }
        n528 = call <vilib>:"Connextion Info.vi"() -> ("Connected"=→"NT Connection":bool)  [unwired: 10 in, 1 out]
      }
      event "CheckList": Double Click {
        # "Shift clears all"
        # "Update symbols on the listbox"
        n529 = event-data() -> ("PlatMods.Shift"=w873:bool, "Row"=w875:i32)  [unwired: 1 in]
        n530 = case shown="True" w873 {
          tunnel: w875 -> [w879 _]
          tunnel: 1 -> [w878 _]
          frame False {
            n531 = property on="CheckList" class="LstBox (strict)"() -> ("Item Symbols"=w877:i32[])  [unwired: 2 in, 2 out]
            n532 = Replace Array Subset(array=w877, new element=w878, index=w879) -> (w876:i32[])
            n533 = property on="CheckList" class="LstBox (strict)"("Item Symbols"=w876) -> ()  [unwired: 2 in, 2 out]
          }
          frame True {
            w880 = 0 ("Top Row")
            n534 = property on="CheckList" class="LstBox (strict)"() -> ("Number of Rows"=w882:u32)  [unwired: 2 in, 2 out]
            n535 = Initialize Array(0, w882) -> (w881:i32[])
            n536 = property on="CheckList" class="LstBox (strict)"("Top Row"=w880, "Value"=w880, "Item Symbols"=w881) -> ()  [unwired: 2 in, 2 out]
          }
        }
      }
      event "CheckList": Key Down {
        # "Update symbols on the listbox\nLeft and right keys check and uncheck"
        n537 = event-data() -> ("VKey"=w885:T28)  [unwired: 1 in]
        n538 = case shown="\"Left\", \"Right\"" w885 {
          selector: w885 -> [w890 _]
          tunnel: eventvkey."Left" ("VKey") -> [w888 _]
          frame "Left", "Right" {
            n539 = Equal?(x=w888, y=w890) -> (x = y?=w889:bool)
            n540 = Select(t=0, s=w889, f=1) -> (s? t:f=w891:i32)
            n541 = property on="CheckList" class="LstBox (strict)"() -> ("Item Symbols"=w894:i32[])  [unwired: 2 in, 2 out]
            n542 = Replace Array Subset(array=w894, new element=w891, index="CheckList") -> (w893:i32[])
            n543 = property on="CheckList" class="LstBox (strict)"("Item Symbols"=w893) -> ()  [unwired: 2 in, 2 out]
          }
          frame Default {
          }
        }
      }
      event "Tree": Double Click {
        n544 = event-data() -> ("PlatMods"=w900:T29, "Tag"=w897:string)  [unwired: 1 in]
        n545 = Unbundle(w900) -> ("Shift"=w899:bool)  [unwired: 4 out]
        n546 = String Subset(string=w897, length (rest)=1 ("length (rest)")) -> (substring=w896:string)  [unwired: 1 in]
        n547 = Not(x=w899) -> (.not. x?=w898:bool)
        n548 = case shown="\"/\"" w896 {
          tunnel: w897 -> [_ w902]
          tunnel: w898 -> [_ w901]
          frame Default {
          }
          frame "/" {
            n549 = call <vilib>:"NT Update Persistence.vi"("Persistence"=w901, "Name"=w902) -> ()  [unwired: 9 in, 1 out]
          }
        }
      }
    }
  }
  n550 = while {
    tunnel: w3 -> [_]
    stop <- FALSE stop-if-true
    # "Maintain LimeLight connection"
    n551 = local read "Enable_Streaming_GUI"() -> (w903:bool)
    n552 = Wait (ms)(milliseconds to wait=u32 1000) -> ()  [unwired: 1 out]
    n553 = case shown="True" w903 {
      frame False {
      }
      frame True {
        w916 = "320x240 MJPEG 22 fps" ("String")
        w910 = "mjpg:http://10.42.65.11:5800"
        w915 = "/CameraPublisher/limelight/"
        # "manually configure the NT for a single LimeLight\ncamera in order to bypass WPILib's camera\nauto-detection which fails when the NTs are refreshed\nafter the code restarts on the roboRIO"
        n554 = Concatenate Strings("ip:http://", "10.42.65.11:5800" ("string")) -> (w918:string)
        n555 = Build Array(w910, w910) -> (w920:string[])
        n556 = Concatenate Strings(w915, "source") -> (w917:string)
        n557 = Concatenate Strings(w915, "description") -> (w921:string)
        n558 = Concatenate Strings(w915, "mode") -> (w922:string)
        n559 = Build Array(w916) -> (w924:string[])
        n560 = Concatenate Strings(w915, "streams") -> (w919:string)
        n561 = Concatenate Strings(w915, "modes") -> (w923:string)
        n562 = call-poly <vilib>:"NT Write Value.vi"("value"=w918, "name"=w917) -> ()  [unwired: 9 in, 1 out]
        n563 = call-poly <vilib>:"NT Write Value.vi"("value"="limelight" ("String"), "name"=w921) -> ()  [unwired: 9 in, 1 out]
        n564 = call-poly <vilib>:"NT Write Value.vi"("value"=w916, "name"=w922) -> ()  [unwired: 9 in, 1 out]
        n565 = call-poly <vilib>:"NT Write Value.vi"("value"=w920, "name"=w919) -> ()  [unwired: 9 in, 1 out]
        n566 = call-poly <vilib>:"NT Write Value.vi"("value"=w924, "name"=w923) -> ()  [unwired: 9 in, 1 out]
      }
    }
  }
  n567 = while {
    tunnel: u16 1741 ("timeout ms (25000)") -> [w926]
    stop <- FALSE stop-if-true
    # "Wait for DS connections"
    n568 = TCP Create Listener(10:w926) -> (0:w925:errorcluster, 3:w927:refnum<k5>)  [unwired: 4 in, 1 out]
    n569 = case shown="No Error" w925 {
      selector: w925 -> [w929 _]
      tunnel: w927 -> [w930 _]
      frame No Error {
        n570 = while {
          tunnel: w930 -> [w933]
          tunnel: w929 -> [w932]
          stop <- FALSE stop-if-true
          n571 = TCP Wait On Listener(8:w932, 11:w933) -> (0:w934:errorcluster, 4:w935:refnum<k5>)  [unwired: 2 in, 3 out]
          n572 = local write "TCP"(w935) -> ()
          n573 = case shown="Error" w934 {
            frame No Error {
            }
            frame Error {
              n574 = Wait (ms)(milliseconds to wait=u32 1000) -> ()  [unwired: 1 out]
            }
          }
        }
      }
      frame Error {
        n575 = Wait (ms)(milliseconds to wait=u32 1000) -> ()  [unwired: 1 out]
      }
    }
  }
  n576 = while {
    shift-right: [w948] -> _
    shift-left: _ -> [w1001]
    shift-right: [w949] -> _
    shift-left: _ -> [w991]
    tunnel: w1 -> [_]
    stop <- FALSE stop-if-true
    # "Dynamic Overlays"
    n577 = To Long Integer(number="Reticule") -> (32bit integer=w982:i32)
    n578 = Wait (ms)(milliseconds to wait=u32 100) -> ()  [unwired: 1 out]
    n579 = Multiply(x=w982, y=2) -> (x*y=w981:i32)
    n580 = control-ref of="WA_Ret_Left"() -> (w962:refnum<vi>)
    n581 = control-ref of="WA_Ret_Right"() -> (w961:refnum<vi>)
    n582 = control-ref of="LL_Ret_Left"() -> (w947:refnum<vi>)
    n583 = control-ref of="LL_Ret_Right"() -> (w946:refnum<vi>)
    n584 = Increment(x=w981) -> (x+1=w968:i32)
    n585 = First Call?() -> (First Call?: T/F=w971:bool)
    n586 = Index Array(array=w991, index #1=w981, index #2=w968) -> (element #1=w985:i32, element #2=w993:i32)
    n587 = Or(x="Up", y="Down") -> (x .or. y?=w997:bool)
    n588 = Or(x="Left", y="Right") -> (x .or. y?=w987:bool)
    n589 = case shown="True" w971 {
      tunnel: [w1012 w1025] -> w948
      tunnel: w1001 -> [w1012 _]
      tunnel: w962 -> [_ w1024]
      tunnel: w961 -> [_ w1023]
      tunnel: w947 -> [_ w1014]
      tunnel: w946 -> [_ w1013]
      frame False {
      }
      frame True {
        n590 = property class="Bool (strict)"(reference=w1024) -> ("Left"=w1022:i32, "Top"=w1021:i32)  [unwired: 1 in, 2 out]
        n591 = property class="Bool (strict)"(reference=w1023) -> ("Left"=w1020:i32, "Top"=w1019:i32)  [unwired: 1 in, 2 out]
        n592 = property class="Bool (strict)"(reference=w1014) -> ("Left"=w1018:i32, "Top"=w1017:i32)  [unwired: 1 in, 2 out]
        n593 = property class="Bool (strict)"(reference=w1013) -> ("Left"=w1016:i32, "Top"=w1015:i32)  [unwired: 1 in, 2 out]
        n594 = Build Array(w1022, w1021, w1020, w1019, w1018, w1017, w1016, w1015) -> (w1025:i32[])
      }
    }
    n595 = Bundle("WA_Ret_Left"=w962, "WA_Ret_Right"=w961, "LL_Ret_Left"=w947, "LL_Ret_Right"=w946) -> (w953:T30)  [unwired: 1 in]
    n596 = Decrement(x=w993) -> (x-1=w1000:i32)
    n597 = Increment(x=w993) -> (x+1=w999:i32)
    n598 = Decrement(x=w985) -> (x-1=w990:i32)
    n599 = Increment(x=w985) -> (x+1=w989:i32)
    n600 = Select(t=w1000, s="Up", f=w999) -> (s? t:f=w998:i32)
    n601 = Select(t=w990, s="Left", f=w989) -> (s? t:f=w988:i32)
    n602 = Select(t=w998, s=w997, f=w993) -> (s? t:f=w967:i32)
    n603 = Select(t=w988, s=w987, f=w985) -> (s? t:f=w986:i32)
    n604 = Replace Array Subset(array=w991, new element #1=w986, index #1=w981, new element #2=w967, index #2=w968) -> (w966:i32[])
    n605 = Current VI's Path() -> (path=w977:path)
    n606 = Strip Path(path=w977) -> (stripped path=w976:path)  [unwired: 1 out]
    n607 = Cluster To Array(cluster=w953) -> (array=w965:refnum<vi>[])
    n608 = Strip Path(path=w976) -> (stripped path=w975:path)  [unwired: 1 out]
    n609 = Array Size(array=w965) -> (size(s)=w964:i32)
    n610 = Build Path(base path=w975, name or relative path=path "reticule positions" ("XML File Path")) -> (appended path=w974:path)
    n611 = Multiply(x=2 ("dimension size"), y=w964) -> (x*y=w970:i32)
    n612 = Initialize Array(0, w970) -> (w960:i32[])
    n613 = call-poly <vilib>:"Read From XML File.vi"("XML File Path"=w974) -> ("error out"=w952:errorcluster, "XML Elements"=w973:string[])  [unwired: 8 in, 1 out]
    n614 = case shown="No Error" w952 {
      tunnel: w973 -> [w1008 _]
      tunnel: w960 -> [w1005 _]
      tunnel: [w1004 i32[] [0, 0, 0, 0, 0, 0, 0, 0, 0, 0, 0, 0] ("value")] -> w950
      frame No Error {
        n615 = Index Array(array=w1008, index=0) -> (element=w1006:string)
        n616 = Unflatten From XML(xml string=w1006, type=w1005) -> (value=w1004:i32[])  [unwired: 1 in, 1 out]
      }
      frame Error {
      }
    }
    n617 = First Call?() -> (First Call?: T/F=w992:bool)
    n618 = Select(t=w950, s=w992, f=w966) -> (s? t:f=w949:i32[])
    n619 = Add(x=w949, y=w948) -> (x+y=w951:i32[])
    n620 = Index Array(array=w951, index #1=0 ("index")) -> (element #1=w957:i32, element #2=w956:i32, element #3=w955:i32, element #4=w954:i32, element #5=w945:i32, element #6=w944:i32, element #7=w943:i32, element #8=w942:i32)  [unwired: 7 in]
    n621 = Unbundle(w953) -> ("WA_Ret_Left"=w958:refnum<vi>, "WA_Ret_Right"=w959:refnum<vi>, "LL_Ret_Left"=w941:refnum<vi>, "LL_Ret_Right"=w940:refnum<vi>)
    n622 = Flatten To XML(6:w949) -> (2:w979:string)
    n623 = call "EdgeTrigger.vi"("Input Signal"="Save") -> ("Rising Edge Trigger"=w938:bool)  [unwired: 2 out]
    n624 = case shown="True" w938 {
      tunnel: w979 -> [_ w1011]
      tunnel: w974 -> [_ w1010]
      frame False {
      }
      frame True {
        n625 = call-poly <vilib>:"Write to XML File.vi"("XML Input"=w1011, "XML File Path"=w1010) -> ()  [unwired: 7 in, 3 out]
      }
    }
    n626 = property class="Bool (strict)"(reference=w958, "Left"=w957, "Top"=w956) -> ()  [unwired: 1 in, 2 out]
    n627 = property class="Bool (strict)"(reference=w959, "Left"=w955, "Top"=w954) -> ()  [unwired: 1 in, 2 out]
    n628 = property class="Bool (strict)"(reference=w941, "Left"=w945, "Top"=w944) -> ()  [unwired: 1 in, 2 out]
    n629 = property class="Bool (strict)"(reference=w940, "Left"=w943, "Top"=w942) -> ()  [unwired: 1 in, 2 out]
  }
  n630 = while {
    tunnel: w10 -> [w1055]
    tunnel: w3 -> [w1039]
    tunnel: w4 -> [w1037]
    stop <- FALSE stop-if-true
    w1026 = u16 0 items=["Stop", "Record", "Playback Panel"] ("Rec Mode")
    # "Camera Feeds"
    n631 = First Call?() -> (First Call?: T/F=w1033:bool)
    n632 = local read "NT Connection"() -> (w1036:bool)
    n633 = call "Timer.vi"("Reset Timer"=w1033) -> ("Time (ms)"=w1032:u32)
    n634 = Greater?(x=w1032, y=u32 5000) -> (0:w1030:bool)
    n635 = Compound Arithmetic op=AND(w1036, "Enable_Streaming_GUI", w1030) -> (w1035:bool)
    n636 = Bundle("Camera Name"="Camera Name", w1039, "Saved DB Images Info"=w1055) -> (w1054:T31)  [unwired: 1 in]
    n637 = control-ref of="Camera Perf"() -> (w1052:refnum<vi>)
    n638 = call <vilib>:"WPI_CameraRead MJPG for Dashboard_2.vi"("Camera Settings"="Camera Settings", "Rec Mode"=w1026, "NT Connection"=w1035, "Capture Info"=w1054, "Image in"=w1037) -> ("perf info"=w1053:cluster{"Bandwidth (Mbps)":dbl, "fps":dbl}, "Active"=w1038:bool, "Image\\ out"=w1056:T3)  [unwired: 4 in]
    n639 = call <vilib>:"WPI_DashboardFormatPerf.vi"("Right Camera Perf"=cluster{"Bandwidth (Mbps)":dbl, "FPS":dbl} {"Bandwidth (Mbps)"=0.0, "FPS"=0.0}, "Performance"=w1053, "String in"=w1052) -> ()  [unwired: 9 in]
    n640 = case shown="True" w1038 {
      tunnel: w1056 -> [w1067 w1070]
      tunnel: [w1067 w1069] -> w1051
      frame False {
        n641 = Wait Until Next ms Multiple(millisecond multiple=u32 500) -> ()  [unwired: 1 out]
      }
      frame True {
        # "image annotation etc."
        n642 = call "IMAQ Clear Overlay"("Image"=w1070) -> ("Image Out"=w1069:T3)  [unwired: 2 in, 8 out]
      }
    }
    n643 = call "IMAQ Rotate"("Angle (degrees)"=sgl 0.0, "Image Src"=w1051) -> ("Image Dst Out"=w1042:T3)  [unwired: 8 in, 1 out]
    n644 = call "IMAQ GetImageSize"("Image"=w1042) -> ("Y Resolution"=w1040:i32, "X Resolution"=w1027:i32)  [unwired: 3 in, 1 out]
    n645 = To Double Precision Float(number=w1027) -> (double precision float=w1049:dbl)
    n646 = To Double Precision Float(number=w1040) -> (double precision float=w1048:dbl)
    n647 = Divide(x=w1049, y=w1048) -> (x/y=w1047:dbl)
    n648 = Less?(x=w1047, y=1.9) -> (x < y?=→"No_Secondary_Camera":bool)
    n649 = case shown="160, Default" w1027 {
      tunnel: "Partial Video Stream" ("Image Name") -> [_ w1066]
      tunnel: [w1058 w1065] -> w1029
      tunnel: w1042 -> [w1058 w1063]
      frame 320 {
        # "wide angle camera found"
      }
      frame 160, Default {
        w1059 = T11 4 items=["Grayscale (U8)", "Grayscale (I16)", "Grayscale (SGL)", "Complex (CSG)", "RGB (U32)", "HSL (U32)", "RGB (U64)"] ("Image Type")
        # "no wide angle camera found"
        n650 = call "IMAQ Create"("Image Name"=w1066, "Image Type"=w1059) -> ("New Image"=w1062:T3)  [unwired: 3 in, 1 out]
        n651 = call "IMAQ SetImageSize"("Y Resolution"=120, "X Resolution"=320, "Image"=w1062) -> ("Image Out"=w1064:T3)  [unwired: 2 in, 1 out]
        n652 = call "IMAQ ImageToImage 2"("Image Src (Small)"=w1063, "Image Src (Large)"=w1064) -> ("Image Dst Out"=w1065:T3)  [unwired: 8 in, 1 out]
      }
    }
    "Combined Camera Feed" <- w1029
  }
  n653 = while {
    stop <- FALSE stop-if-true
    # "Error Message Handling"
    n654 = property on="Actuator Testing" class="Ring (strict)"() -> ("RingText.Text"=w1140:string)  [unwired: 2 in, 2 out]
    n655 = local read "Arm_Motor_Over_Current"() -> (w1081:bool)
    n656 = local read "Master_Safety_Override_1"() -> (w1111:bool)
    n657 = local read "Arm_Calibrate_Wheels_GUI"() -> (w1160:bool)
    n658 = local read "Arm_Calibrate_Joysticks"() -> (w1130:bool)
    n659 = local read "Swerve_Shifter_Failure"() -> (w1121:bool)
    n660 = local read "CAN_Bus_Fault_GUI"() -> (w1127:bool)
    n661 = Wait (ms)(milliseconds to wait=u32 200) -> ()  [unwired: 1 out]
    n662 = local read "Gripper_Overheating"() -> (w1074:bool)
    n663 = local read "Gripper_Motor_Fault"() -> (w1073:bool)
    n664 = local read "Swerve_Azimuth_Fault"() -> (w1164:bool)
    n665 = local read "Home_Wheels_GUI"() -> (w1113:bool)
    n666 = Not Equal?(x=w1140, y="No_Test") -> (x != y?=w1147:bool)
    n667 = local read "Swerve_Overheating"() -> (w1173:bool)
    n668 = local read "Unlock_Arm_Joints"() -> (w1092:bool)
    n669 = local read "Arm_Overheating"() -> (w1103:bool)
    n670 = local read "Super_Test_Mode_GUI"() -> (w1181:bool)
    n671 = call <vilib>:"Space Constant.vi"() -> ("String"=w1138:string)
    n672 = local read "Swerve_Drive_Fault"() -> (w1096:bool)
    n673 = local read "Auto_Test_Mode_GUI"() -> (w1152:bool)
    n674 = local read "Arm_Motor_Fault"() -> (w1082:bool)
    n675 = local read "Arm_Calibrate_Arm"() -> (w1100:bool)
    n676 = local read "IMU_Failure_GUI"() -> (w1144:bool)
    n677 = local read "Electrical_Fault_GUI"() -> (w1135:bool)
    n678 = local read "Vision_Fault_GUI"() -> (w1108:bool)
    n679 = local read "Pressure_Vent_GUI"() -> (w1169:bool)
    n680 = local read "Simulate_Arm"() -> (w1088:bool)
    n681 = local read "Auto_Error_GUI"() -> (w1157:bool)
    n682 = Search and Replace String(replace all?=TRUE ("replace all? (F)"), input string=w1140, search string="_", replace string=w1138) -> (result string=w1141:string)  [unwired: 4 in, 3 out]
    n683 = local read "Slow_Loop"() -> (w1176:bool)
    n684 = Concatenate Strings("testing " ("string"), w1141) -> (w1150:string)
    n685 = Bundle("homing the wheels", "Home_Wheels_GUI"=w1113, 60.0) -> (w1112:cluster{string, "Home_Wheels_GUI":bool, dbl})  [unwired: 1 in]
    n686 = Bundle("gripper motor has failed", "Gripper_Motor_Fault"=w1073, 10.0) -> (w1071:cluster{string, "Gripper_Motor_Fault":bool, dbl})  [unwired: 1 in]
    n687 = Bundle("arm motor siezed, arm is locked out", "Arm_Motor_Over_Current"=w1081, 10.0) -> (w1079:T32)  [unwired: 1 in]
    n688 = Bundle("gripper is overheating", "Gripper_Overheating"=w1074, 60.0) -> (w1072:cluster{string, "Gripper_Overheating":bool, dbl})  [unwired: 1 in]
    n689 = Bundle("arm overheating", "Arm_Overheating"=w1103, 60.0) -> (w1104:cluster{string, "Arm_Overheating":bool, dbl})  [unwired: 1 in]
    n690 = Bundle("swerve shifter failure, forced into low gear", "Swerve_Shifter_Failure"=w1121, 600.0) -> (w1120:T33)  [unwired: 1 in]
    n691 = Bundle("Lime Light failure", "Vision_Fault_GUI"=w1108, 600.0) -> (w1107:cluster{string, "Vision_Fault_GUI":bool, dbl})  [unwired: 1 in]
    n692 = Bundle("swerve drive failure", "Swerve_Drive_Fault"=w1096, 600.0) -> (w1095:cluster{string, "Swerve_Drive_Fault":bool, dbl})  [unwired: 1 in]
    n693 = Bundle("arm joints are now unlocked when disabled", "Unlock_Arm_Joints"=w1092, 60.0) -> (w1091:cluster{string, "Unlock_Arm_Joints":bool, dbl})  [unwired: 1 in]
    n694 = Bundle("arm motor failure, arm is locked out", "Arm_Motor_Fault"=w1082, 10.0) -> (w1080:cluster{string, "Arm_Motor_Fault":bool, dbl})  [unwired: 1 in]
    n695 = Bundle("safeties disengaged", "Master_Safety_Override_1"=w1111, 10.0) -> (w1185:T34)  [unwired: 1 in]
    n696 = Bundle("disabled test mode", "Super_Test_Mode_GUI"=w1181, 10.0) -> (w1184:cluster{string, "Super_Test_Mode_GUI":bool, dbl})  [unwired: 1 in]
    n697 = Bundle("control latency too high", "Slow_Loop"=w1176, 60.0) -> (w1177:cluster{string, "Slow_Loop":bool, dbl})  [unwired: 1 in]
    n698 = Bundle("drive train overheating", "Swerve_Overheating"=w1173, 60.0) -> (w1172:cluster{string, "Swerve_Overheating":bool, dbl})  [unwired: 1 in]
    n699 = Bundle("pressure venting", "Pressure_Vent_GUI"=w1169, 600.0) -> (w1168:cluster{string, "Pressure_Vent_GUI":bool, dbl})  [unwired: 1 in]
    n700 = Bundle("swerve azimuth failure", "Swerve_Azimuth_Fault"=w1164, 600.0) -> (w1165:T35)  [unwired: 1 in]
    n701 = Bundle("ready to calibrate swerve modules", "Arm_Calibrate_Wheels_GUI"=w1160, 10.0) -> (w1161:T36)  [unwired: 1 in]
    n702 = Bundle("autonomous play failure", "Auto_Error_GUI"=w1157, 10.0) -> (w1156:cluster{string, "Auto_Error_GUI":bool, dbl})  [unwired: 1 in]
    n703 = Bundle("autonomous test mode", "Auto_Test_Mode_GUI"=w1152, 10.0) -> (w1153:cluster{string, "Auto_Test_Mode_GUI":bool, dbl})  [unwired: 1 in]
    n704 = Bundle(w1150, w1147, 10.0) -> (w1146:cluster{string, bool, dbl})  [unwired: 1 in]
    n705 = Bundle("IMU failure, auto-targeting disabled", "IMU_Failure_GUI"=w1144, 600.0) -> (w1142:cluster{string, "IMU_Failure_GUI":bool, dbl})  [unwired: 1 in]
    n706 = Bundle("simulating the arm", "Simulate_Arm"=w1088, 60.0) -> (w1087:cluster{string, "Simulate_Arm":bool, dbl})  [unwired: 1 in]
    n707 = Bundle("electrical bus fault, power down", "Electrical_Fault_GUI"=w1135, 60.0) -> (w1134:T37)  [unwired: 1 in]
    n708 = Bundle("ready to calibrate joysticks, wait ten seconds after pressing calibrate", "Arm_Calibrate_Joysticks"=w1130, 10.0) -> (w1131:T38)  [unwired: 1 in]
    n709 = Bundle("CAN bus fault, check wiring", "CAN_Bus_Fault_GUI"=w1127, 60.0) -> (w1129:cluster{string, "CAN_Bus_Fault_GUI":bool, dbl})  [unwired: 1 in]
    n710 = Bundle("ready to calibrate arm encoders", "Arm_Calibrate_Arm"=w1100, 10.0) -> (w1099:cluster{string, "Arm_Calibrate_Arm":bool, dbl})  [unwired: 1 in]
    n711 = local read "Audible_Warnings_Enabled_GUI"() -> (w1119:bool)
    n712 = Build Array(w1185, w1184, w1177, w1172, w1168, w1165, w1161, w1156, w1153, w1146, w1142, w1134, w1131, w1129, w1120, w1112, w1107, w1104, w1099, w1095, w1091, w1087, w1080, w1079, w1072, w1071) -> (w1183:T39)
    n713 = call "EdgeTrigger.vi"("Input Signal"=w1119) -> ("All Edge Trigger"=w1118:bool)  [unwired: 2 out]
    n714 = call "ErrorMessageBuilder.vi"("Errors"=w1183, "Reset Error History"=w1118) -> ("Combined Error String"=w1124:string)
    n715 = Not Equal?(x="", y=w1124) -> (x != y?=w1125:bool)
    n716 = Compound Arithmetic op=AND(w1119, w1125) -> (w1117:bool)
    n717 = case shown="True" w1117 {
      tunnel: w1124 -> [_ w1192]
      frame False {
      }
      frame True {
        n718 = call "TextToSpeech.vi"("Text To Be Spoken"=w1192) -> ()  [unwired: 9 in, 2 out]
      }
    }
    n719 = case shown="True" w1125 {
      tunnel: w1124 -> [_ w1191]
      frame False {
      }
      frame True {
        "Combined Error String" <- w1191
      }
    }
  }
